vi "DalyLab_Oscilloscope_DAQ_v1.0.vi"() -> ()   [LabVIEW 2017]
uses:
  897ebd14-b167-4137-bf33-77dfcdb94355.vi
  <vilib>/Utility/file.llb/Write Delimited Spreadsheet (DBL).vi
  <instrlib>/Keysight InfiniiVision/Keysight InfiniiVision.lvlib
panel:
  in  "Tab Control":T1(tab)
  in  "Frequency Sweep":bool
  out "SWEEP IN PROGRESS":bool
  in  "Amplitude (Vpp)":dbl=5.0 format="%#_13g"
  in  "Initial Frequency (Hz)":dbl=20000.0 format="%#_13g"
  in  "Stop Frequency (Hz)":dbl=30000.0 format="%#_13g"
  in  "Freq. Increments (Hz)":dbl=1000.0 format="%#_13g"
  in  "Acq. per Freq.":i32=1
  out "Sine Freq (Hz)":dbl format="%#_13g"
  in  "Delay (ms)":dbl=1000.0 format="%#_13g"
  in  "Pulse Generation":bool
  out "PULSING IN PROGRESS":bool
  in  "Pulse Width (s)":dbl=1e-06 format="%#_13g"
  in  "Rate (pulse/second)":dbl=1.0 format="%#_13g"
  in  "Pulse Amplitude (V)":dbl=5.0 format="%#_13g"
  in  "Number of Pulses":i32=30
  in  "Acquisition":bool
  in  "Stop Acquisition":bool
  out "ACQUISITION IN PROGRESS":bool
  out "Channel 2":dbl[](graph)
  out "EVENT COUNTER":dbl
  out "Log":string caption="LOG"
  out "Channel 1":dbl[](graph)
  in  "Acq. Start Time (s)":dbl=-0.0008
  in  "Horizontal Scale (s/div)":dbl=0.0002
  in  "Channel 2 Atten.":dbl=1.0 format="%#_13g"
  in  "Channel 1 Atten.":dbl=1.0 format="%#_13g"
  in  "Channel 2 Offset (V)":dbl
  in  "Channel 2 Scale (V/div)":dbl=0.05
  in  "Channel 1 Offset (V)":dbl
  in  "Channel 1 Scale (V/div)":dbl=1.0
  in  "Trigger Edge Level (V)":dbl=0.05
  in  "Trigger Edge Source":u16(ring) items=["Channel1", "Channel2"]
  in  "Test Operator":string
  out "File Path":path
  in  "File Name":string
  in  "Save Directory":path
  in  "Oscilloscope VISA address":string="USB0::0x0957::0x1797::MY56271380::0::INSTR" caption="Oscilloscope VISA Address"
  in  "Waveform Size":i32=50000
  out "Test Type":i32
  # "OSCILLOSCOPE CONFIGURATION"
  # "TESTING"
  # "SETUP"
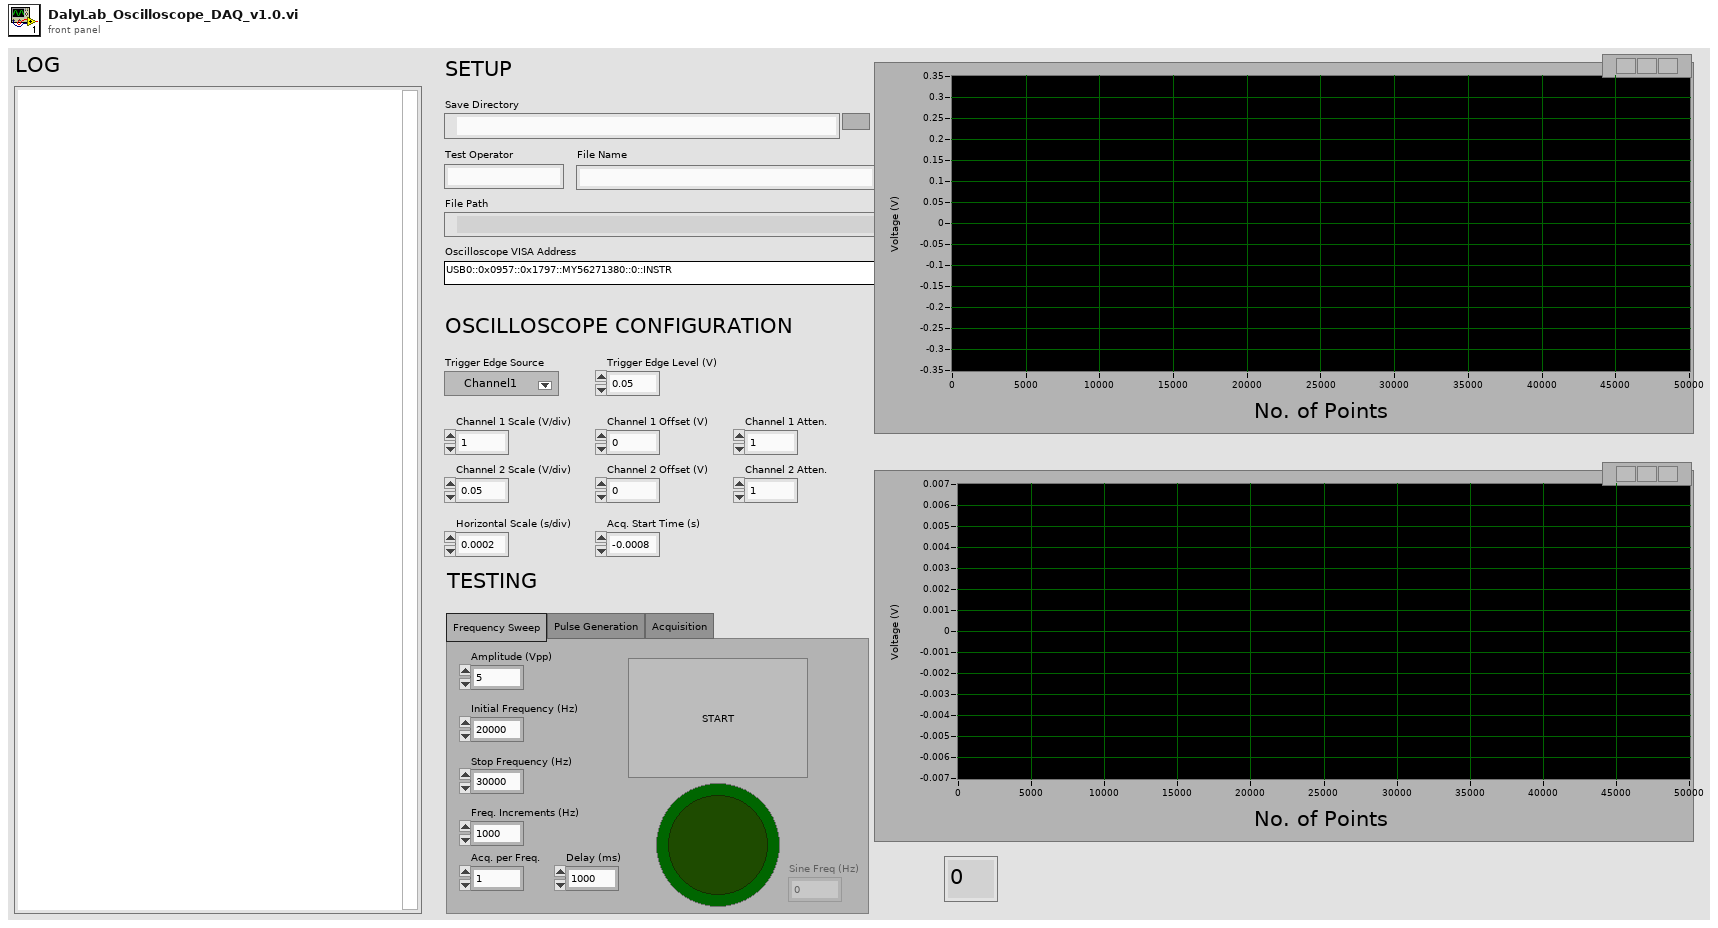
[diagram p1: front panel]
types:
  T1 = enum32{"Frequency Sweep", "Pulse Generation", "Acquisition"}
  T2 = enum16{"open", "replace", "create", "open or create", "replace or create", "replace or create with confirmation"}
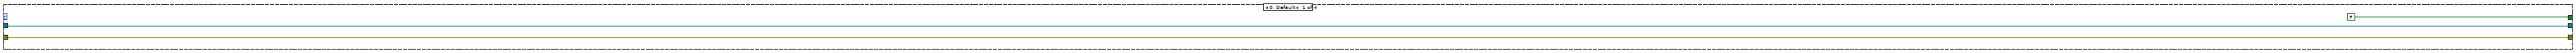
[diagram p5: hidden frame]
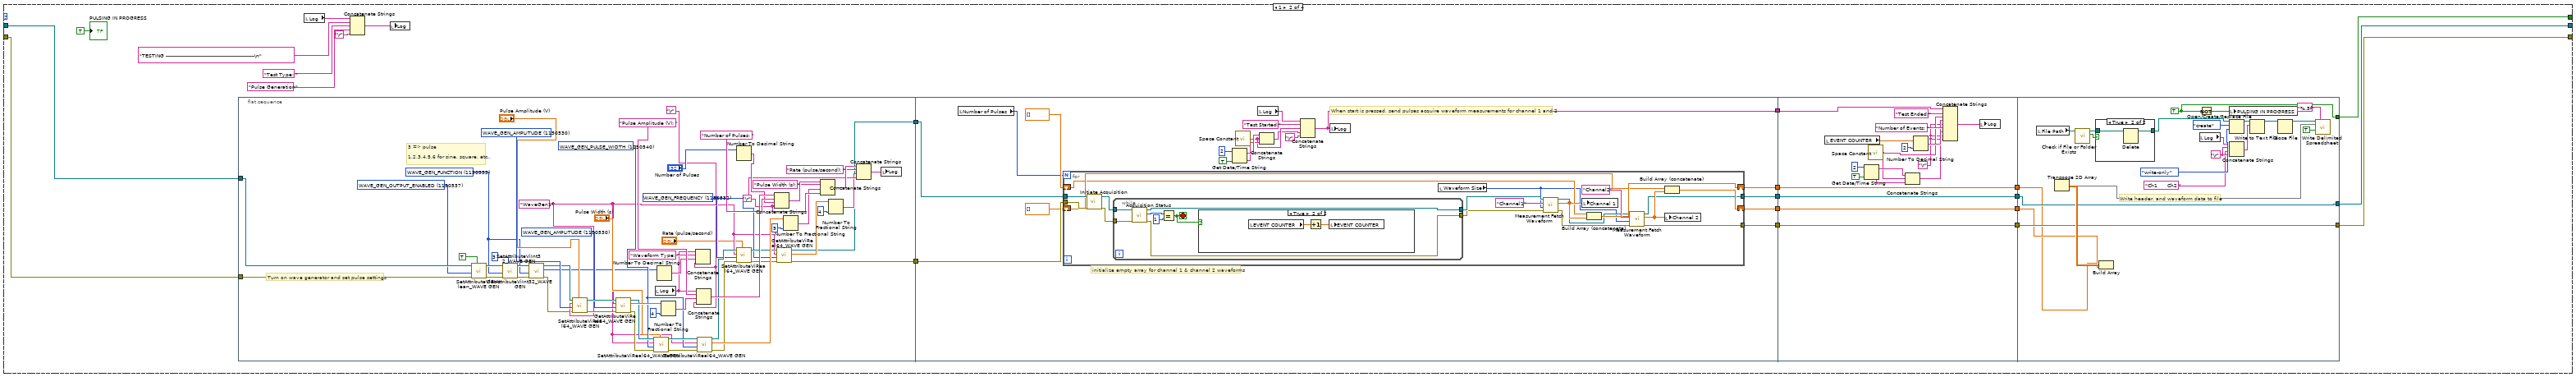
[diagram p6: hidden frame]
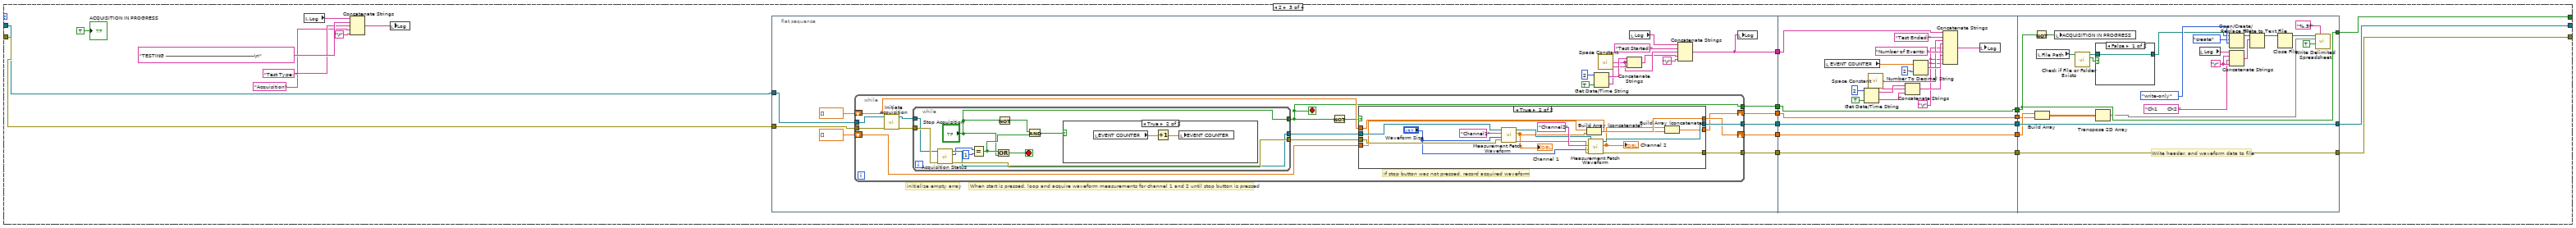
[diagram p9: hidden frame]
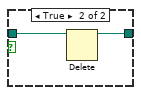
[diagram p12: hidden frame]
diagram:
  w2 = u32 1150537 items=["ARBITRARY_INTERPOLATION"=1150411, "MODULATION_ENABLED"=1150554, "TRACKING_AMPLITUDE"=1150527, "TRACKING_ENABLED"=1150526, "TRACKING_FREQUENCY"=1150528, "WAVE_GEN_ARBITRARY_INTERPOLATION"=1150543, "WAVE_GEN_OUTPUT_ENABLED"=1150537, "WAVE_GEN_OUTPUT_INVERTED"=1150545] ("AttributeID")
  w9 = "\r"
  w18 = "\r"
  w22 = "\r"
  w50 = u32 1250004 items=["ACQUISITION_START_TIME"=1250109, "CHANNEL_PROBE_SKEW"=1150030, "CHANNEL_SCALE"=1150032, "EXTERNAL_PROBE_ATTENUATION"=1150012, "EXTERNAL_RANGE"=1150015, "GLITCH_WIDTH"=1250401, "HORZ_TIME_PER_RECORD"=1250007, "INPUT_IMPEDANCE"=1250103, "INTEGRATE_INPUT_OFFSET"=1150360, "MAX_INPUT_FREQUENCY"=1250006, "MEAS_HIGH_REF"=1250607, "MEAS_LOW_REF"=1250608, "MEAS_MID_REF"=1250609, "PROBE_ATTENUATION"=1250004, "RUNT_HIGH_THRESHOLD"=1250301, "RUNT_LOW_THRESHOLD"=1250302, "TIMEBASE_HORIZONTAL_SCALE"=1150111, "TIMEBASE_WINDOW_HORIZONTAL_SCALE"=1150115, "TIMEBASE_WINDOW_POSITION"=1150113, "TIMEBASE_WINDOW_RANGE"=1150114, "TRIGGER_DELAY_TIME"=1150265, "TRIGGER_EDGE_BURST_IDLE_TIME"=1150248, "TRIGGER_GLITCH_LEVEL"=1150134, "TRIGGER_HOLDOFF"=1250016, "TRIGGER_LEVEL"=1250017, "TRIGGER_PATTERN_MAX_DURATION"=1150166, "TRIGGER_PATTERN_MIN_WIDTH"=1150158, "TRIGGER_RUNT_QUALIFIER_TIME"=1150191, "TRIGGER_SETUP_AND_HOLD_HOLD_TIME"=1150251, "TRIGGER_SETUP_AND_HOLD_SETUP_TIME"=1150252, "TRIGGER_TRANSITION_QUALIFIER_TIME"=1150257, "TRIGGER_TRANSITION_THRESHOLD_HIGH"=1150428, "TRIGGER_TRANSITION_THRESHOLD_LOW"=1150429, "TRIGGER_WIDTH_THRESHOLD_HIGH"=1150198, "TRIGGER_WIDTH_THRESHOLD_LOW"=1150199, "VERTICAL_OFFSET"=1250002, "VERTICAL_RANGE"=1250001, "WIDTH_HIGH_THRESHOLD"=1250502, "WIDTH_LOW_THRESHOLD"=1250501] ("AttributeID")
  w51 = "Channel2"
  w70 = "Channel1"
  w69 = u32 1250004 items=["ACQUISITION_START_TIME"=1250109, "CHANNEL_PROBE_SKEW"=1150030, "CHANNEL_SCALE"=1150032, "EXTERNAL_PROBE_ATTENUATION"=1150012, "EXTERNAL_RANGE"=1150015, "GLITCH_WIDTH"=1250401, "HORZ_TIME_PER_RECORD"=1250007, "INPUT_IMPEDANCE"=1250103, "INTEGRATE_INPUT_OFFSET"=1150360, "MAX_INPUT_FREQUENCY"=1250006, "MEAS_HIGH_REF"=1250607, "MEAS_LOW_REF"=1250608, "MEAS_MID_REF"=1250609, "PROBE_ATTENUATION"=1250004, "RUNT_HIGH_THRESHOLD"=1250301, "RUNT_LOW_THRESHOLD"=1250302, "TIMEBASE_HORIZONTAL_SCALE"=1150111, "TIMEBASE_WINDOW_HORIZONTAL_SCALE"=1150115, "TIMEBASE_WINDOW_POSITION"=1150113, "TIMEBASE_WINDOW_RANGE"=1150114, "TRIGGER_DELAY_TIME"=1150265, "TRIGGER_EDGE_BURST_IDLE_TIME"=1150248, "TRIGGER_GLITCH_LEVEL"=1150134, "TRIGGER_HOLDOFF"=1250016, "TRIGGER_LEVEL"=1250017, "TRIGGER_PATTERN_MAX_DURATION"=1150166, "TRIGGER_PATTERN_MIN_WIDTH"=1150158, "TRIGGER_RUNT_QUALIFIER_TIME"=1150191, "TRIGGER_SETUP_AND_HOLD_HOLD_TIME"=1150251, "TRIGGER_SETUP_AND_HOLD_SETUP_TIME"=1150252, "TRIGGER_TRANSITION_QUALIFIER_TIME"=1150257, "TRIGGER_TRANSITION_THRESHOLD_HIGH"=1150428, "TRIGGER_TRANSITION_THRESHOLD_LOW"=1150429, "TRIGGER_WIDTH_THRESHOLD_HIGH"=1150198, "TRIGGER_WIDTH_THRESHOLD_LOW"=1150199, "VERTICAL_OFFSET"=1250002, "VERTICAL_RANGE"=1250001, "WIDTH_HIGH_THRESHOLD"=1250502, "WIDTH_LOW_THRESHOLD"=1250501] ("AttributeID")
  w81 = "Channel2"
  w84 = u32 1250002 items=["ACQUISITION_START_TIME"=1250109, "CHANNEL_PROBE_SKEW"=1150030, "CHANNEL_SCALE"=1150032, "EXTERNAL_PROBE_ATTENUATION"=1150012, "EXTERNAL_RANGE"=1150015, "GLITCH_WIDTH"=1250401, "HORZ_TIME_PER_RECORD"=1250007, "INPUT_IMPEDANCE"=1250103, "INTEGRATE_INPUT_OFFSET"=1150360, "MAX_INPUT_FREQUENCY"=1250006, "MEAS_HIGH_REF"=1250607, "MEAS_LOW_REF"=1250608, "MEAS_MID_REF"=1250609, "PROBE_ATTENUATION"=1250004, "RUNT_HIGH_THRESHOLD"=1250301, "RUNT_LOW_THRESHOLD"=1250302, "TIMEBASE_HORIZONTAL_SCALE"=1150111, "TIMEBASE_WINDOW_HORIZONTAL_SCALE"=1150115, "TIMEBASE_WINDOW_POSITION"=1150113, "TIMEBASE_WINDOW_RANGE"=1150114, "TRIGGER_DELAY_TIME"=1150265, "TRIGGER_EDGE_BURST_IDLE_TIME"=1150248, "TRIGGER_GLITCH_LEVEL"=1150134, "TRIGGER_HOLDOFF"=1250016, "TRIGGER_LEVEL"=1250017, "TRIGGER_PATTERN_MAX_DURATION"=1150166, "TRIGGER_PATTERN_MIN_WIDTH"=1150158, "TRIGGER_RUNT_QUALIFIER_TIME"=1150191, "TRIGGER_SETUP_AND_HOLD_HOLD_TIME"=1150251, "TRIGGER_SETUP_AND_HOLD_SETUP_TIME"=1150252, "TRIGGER_TRANSITION_QUALIFIER_TIME"=1150257, "TRIGGER_TRANSITION_THRESHOLD_HIGH"=1150428, "TRIGGER_TRANSITION_THRESHOLD_LOW"=1150429, "TRIGGER_WIDTH_THRESHOLD_HIGH"=1150198, "TRIGGER_WIDTH_THRESHOLD_LOW"=1150199, "VERTICAL_OFFSET"=1250002, "VERTICAL_RANGE"=1250001, "WIDTH_HIGH_THRESHOLD"=1250502, "WIDTH_LOW_THRESHOLD"=1250501] ("AttributeID")
  w85 = u32 1250002 items=["ACQUISITION_START_TIME"=1250109, "CHANNEL_PROBE_SKEW"=1150030, "CHANNEL_SCALE"=1150032, "EXTERNAL_PROBE_ATTENUATION"=1150012, "EXTERNAL_RANGE"=1150015, "GLITCH_WIDTH"=1250401, "HORZ_TIME_PER_RECORD"=1250007, "INPUT_IMPEDANCE"=1250103, "INTEGRATE_INPUT_OFFSET"=1150360, "MAX_INPUT_FREQUENCY"=1250006, "MEAS_HIGH_REF"=1250607, "MEAS_LOW_REF"=1250608, "MEAS_MID_REF"=1250609, "PROBE_ATTENUATION"=1250004, "RUNT_HIGH_THRESHOLD"=1250301, "RUNT_LOW_THRESHOLD"=1250302, "TIMEBASE_HORIZONTAL_SCALE"=1150111, "TIMEBASE_WINDOW_HORIZONTAL_SCALE"=1150115, "TIMEBASE_WINDOW_POSITION"=1150113, "TIMEBASE_WINDOW_RANGE"=1150114, "TRIGGER_DELAY_TIME"=1150265, "TRIGGER_EDGE_BURST_IDLE_TIME"=1150248, "TRIGGER_GLITCH_LEVEL"=1150134, "TRIGGER_HOLDOFF"=1250016, "TRIGGER_LEVEL"=1250017, "TRIGGER_PATTERN_MAX_DURATION"=1150166, "TRIGGER_PATTERN_MIN_WIDTH"=1150158, "TRIGGER_RUNT_QUALIFIER_TIME"=1150191, "TRIGGER_SETUP_AND_HOLD_HOLD_TIME"=1150251, "TRIGGER_SETUP_AND_HOLD_SETUP_TIME"=1150252, "TRIGGER_TRANSITION_QUALIFIER_TIME"=1150257, "TRIGGER_TRANSITION_THRESHOLD_HIGH"=1150428, "TRIGGER_TRANSITION_THRESHOLD_LOW"=1150429, "TRIGGER_WIDTH_THRESHOLD_HIGH"=1150198, "TRIGGER_WIDTH_THRESHOLD_LOW"=1150199, "VERTICAL_OFFSET"=1250002, "VERTICAL_RANGE"=1250001, "WIDTH_HIGH_THRESHOLD"=1250502, "WIDTH_LOW_THRESHOLD"=1250501] ("AttributeID")
  w103 = u32 1150032 items=["ACQUISITION_SEGMENTEDMEMORY_TIME_TAG"=1150140, "ACQUISITION_START_TIME"=1250109, "CHANNEL_PROBE_SKEW"=1150030, "CHANNEL_SCALE"=1150032, "DVM_CURRENT"=1150440, "DVM_FREQUENCY"=1150442, "EXTERNAL_PROBE_ATTENUATION"=1150012, "EXTERNAL_PROBE_SENSE"=1150013, "EXTERNAL_RANGE"=1150015, "GLITCH_WIDTH"=1250401, "HORZ_SAMPLE_RATE"=1250010, "HORZ_TIME_PER_RECORD"=1250007, "INPUT_IMPEDANCE"=1250103, "INTEGRATE_INPUT_OFFSET"=1150360, "MAX_INPUT_FREQUENCY"=1250006, "MEAS_HIGH_REF"=1250607, "MEAS_LOW_REF"=1250608, "MEAS_MID_REF"=1250609, "PROBE_ATTENUATION"=1250004, "PROBE_SENSE_VALUE"=1250108, "RUNT_HIGH_THRESHOLD"=1250301, "RUNT_LOW_THRESHOLD"=1250302, "TIMEBASE_HORIZONTAL_SCALE"=1150111, "TIMEBASE_WINDOW_HORIZONTAL_SCALE"=1150115, "TIMEBASE_WINDOW_POSITION"=1150113, "TIMEBASE_WINDOW_RANGE"=1150114, "TRIGGER_DELAY_TIME"=1150265, "TRIGGER_EDGE_BURST_IDLE_TIME"=1150248, "TRIGGER_GLITCH_LEVEL"=1150134, "TRIGGER_HOLDOFF"=1250016, "TRIGGER_LEVEL"=1250017, "TRIGGER_PATTERN_MAX_DURATION"=1150166, "TRIGGER_PATTERN_MIN_WIDTH"=1150158, "TRIGGER_RUNT_QUALIFIER_TIME"=1150191, "TRIGGER_SETUP_AND_HOLD_HOLD_TIME"=1150251, "TRIGGER_SETUP_AND_HOLD_SETUP_TIME"=1150252, "TRIGGER_TRANSITION_QUALIFIER_TIME"=1150257, "TRIGGER_TRANSITION_THRESHOLD_HIGH"=1150428, "TRIGGER_TRANSITION_THRESHOLD_LOW"=1150429, "TRIGGER_WIDTH_THRESHOLD_HIGH"=1150198, "TRIGGER_WIDTH_THRESHOLD_LOW"=1150199, "VERTICAL_OFFSET"=1250002, "VERTICAL_RANGE"=1250001, "WAVEFORM_X_INCREMENT"=1150143, "WAVEFORM_X_ORIGIN"=1150147, "WAVEFORM_Y_INCREMENT"=1150144, "WAVEFORM_Y_ORIGIN"=1150148, "WIDTH_HIGH_THRESHOLD"=1250502, "WIDTH_LOW_THRESHOLD"=1250501] ("AttributeID")
  w104 = u32 1150032 items=["ACQUISITION_SEGMENTEDMEMORY_TIME_TAG"=1150140, "ACQUISITION_START_TIME"=1250109, "CHANNEL_PROBE_SKEW"=1150030, "CHANNEL_SCALE"=1150032, "DVM_CURRENT"=1150440, "DVM_FREQUENCY"=1150442, "EXTERNAL_PROBE_ATTENUATION"=1150012, "EXTERNAL_PROBE_SENSE"=1150013, "EXTERNAL_RANGE"=1150015, "GLITCH_WIDTH"=1250401, "HORZ_SAMPLE_RATE"=1250010, "HORZ_TIME_PER_RECORD"=1250007, "INPUT_IMPEDANCE"=1250103, "INTEGRATE_INPUT_OFFSET"=1150360, "MAX_INPUT_FREQUENCY"=1250006, "MEAS_HIGH_REF"=1250607, "MEAS_LOW_REF"=1250608, "MEAS_MID_REF"=1250609, "PROBE_ATTENUATION"=1250004, "PROBE_SENSE_VALUE"=1250108, "RUNT_HIGH_THRESHOLD"=1250301, "RUNT_LOW_THRESHOLD"=1250302, "TIMEBASE_HORIZONTAL_SCALE"=1150111, "TIMEBASE_WINDOW_HORIZONTAL_SCALE"=1150115, "TIMEBASE_WINDOW_POSITION"=1150113, "TIMEBASE_WINDOW_RANGE"=1150114, "TRIGGER_DELAY_TIME"=1150265, "TRIGGER_EDGE_BURST_IDLE_TIME"=1150248, "TRIGGER_GLITCH_LEVEL"=1150134, "TRIGGER_HOLDOFF"=1250016, "TRIGGER_LEVEL"=1250017, "TRIGGER_PATTERN_MAX_DURATION"=1150166, "TRIGGER_PATTERN_MIN_WIDTH"=1150158, "TRIGGER_RUNT_QUALIFIER_TIME"=1150191, "TRIGGER_SETUP_AND_HOLD_HOLD_TIME"=1150251, "TRIGGER_SETUP_AND_HOLD_SETUP_TIME"=1150252, "TRIGGER_TRANSITION_QUALIFIER_TIME"=1150257, "TRIGGER_TRANSITION_THRESHOLD_HIGH"=1150428, "TRIGGER_TRANSITION_THRESHOLD_LOW"=1150429, "TRIGGER_WIDTH_THRESHOLD_HIGH"=1150198, "TRIGGER_WIDTH_THRESHOLD_LOW"=1150199, "VERTICAL_OFFSET"=1250002, "VERTICAL_RANGE"=1250001, "WAVEFORM_X_INCREMENT"=1150143, "WAVEFORM_X_ORIGIN"=1150147, "WAVEFORM_Y_INCREMENT"=1150144, "WAVEFORM_Y_ORIGIN"=1150148, "WIDTH_HIGH_THRESHOLD"=1250502, "WIDTH_LOW_THRESHOLD"=1250501] ("AttributeID")
  w102 = "Channel2"
  w28 = FALSE
  w119 = u32 1250109 items=["ACQUISITION_START_TIME"=1250109, "CHANNEL_PROBE_SKEW"=1150030, "CHANNEL_SCALE"=1150032, "EXTERNAL_PROBE_ATTENUATION"=1150012, "EXTERNAL_RANGE"=1150015, "GLITCH_WIDTH"=1250401, "HORZ_TIME_PER_RECORD"=1250007, "INPUT_IMPEDANCE"=1250103, "INTEGRATE_INPUT_OFFSET"=1150360, "MAX_INPUT_FREQUENCY"=1250006, "MEAS_HIGH_REF"=1250607, "MEAS_LOW_REF"=1250608, "MEAS_MID_REF"=1250609, "PROBE_ATTENUATION"=1250004, "RUNT_HIGH_THRESHOLD"=1250301, "RUNT_LOW_THRESHOLD"=1250302, "TIMEBASE_HORIZONTAL_SCALE"=1150111, "TIMEBASE_WINDOW_HORIZONTAL_SCALE"=1150115, "TIMEBASE_WINDOW_POSITION"=1150113, "TIMEBASE_WINDOW_RANGE"=1150114, "TRIGGER_DELAY_TIME"=1150265, "TRIGGER_EDGE_BURST_IDLE_TIME"=1150248, "TRIGGER_GLITCH_LEVEL"=1150134, "TRIGGER_HOLDOFF"=1250016, "TRIGGER_LEVEL"=1250017, "TRIGGER_PATTERN_MAX_DURATION"=1150166, "TRIGGER_PATTERN_MIN_WIDTH"=1150158, "TRIGGER_RUNT_QUALIFIER_TIME"=1150191, "TRIGGER_SETUP_AND_HOLD_HOLD_TIME"=1150251, "TRIGGER_SETUP_AND_HOLD_SETUP_TIME"=1150252, "TRIGGER_TRANSITION_QUALIFIER_TIME"=1150257, "TRIGGER_TRANSITION_THRESHOLD_HIGH"=1150428, "TRIGGER_TRANSITION_THRESHOLD_LOW"=1150429, "TRIGGER_WIDTH_THRESHOLD_HIGH"=1150198, "TRIGGER_WIDTH_THRESHOLD_LOW"=1150199, "VERTICAL_OFFSET"=1250002, "VERTICAL_RANGE"=1250001, "WIDTH_HIGH_THRESHOLD"=1250502, "WIDTH_LOW_THRESHOLD"=1250501] ("AttributeID")
  w121 = u32 1250109 items=["ACQUISITION_START_TIME"=1250109, "CHANNEL_PROBE_SKEW"=1150030, "CHANNEL_SCALE"=1150032, "EXTERNAL_PROBE_ATTENUATION"=1150012, "EXTERNAL_RANGE"=1150015, "GLITCH_WIDTH"=1250401, "HORZ_TIME_PER_RECORD"=1250007, "INPUT_IMPEDANCE"=1250103, "INTEGRATE_INPUT_OFFSET"=1150360, "MAX_INPUT_FREQUENCY"=1250006, "MEAS_HIGH_REF"=1250607, "MEAS_LOW_REF"=1250608, "MEAS_MID_REF"=1250609, "PROBE_ATTENUATION"=1250004, "RUNT_HIGH_THRESHOLD"=1250301, "RUNT_LOW_THRESHOLD"=1250302, "TIMEBASE_HORIZONTAL_SCALE"=1150111, "TIMEBASE_WINDOW_HORIZONTAL_SCALE"=1150115, "TIMEBASE_WINDOW_POSITION"=1150113, "TIMEBASE_WINDOW_RANGE"=1150114, "TRIGGER_DELAY_TIME"=1150265, "TRIGGER_EDGE_BURST_IDLE_TIME"=1150248, "TRIGGER_GLITCH_LEVEL"=1150134, "TRIGGER_HOLDOFF"=1250016, "TRIGGER_LEVEL"=1250017, "TRIGGER_PATTERN_MAX_DURATION"=1150166, "TRIGGER_PATTERN_MIN_WIDTH"=1150158, "TRIGGER_RUNT_QUALIFIER_TIME"=1150191, "TRIGGER_SETUP_AND_HOLD_HOLD_TIME"=1150251, "TRIGGER_SETUP_AND_HOLD_SETUP_TIME"=1150252, "TRIGGER_TRANSITION_QUALIFIER_TIME"=1150257, "TRIGGER_TRANSITION_THRESHOLD_HIGH"=1150428, "TRIGGER_TRANSITION_THRESHOLD_LOW"=1150429, "TRIGGER_WIDTH_THRESHOLD_HIGH"=1150198, "TRIGGER_WIDTH_THRESHOLD_LOW"=1150199, "VERTICAL_OFFSET"=1250002, "VERTICAL_RANGE"=1250001, "WIDTH_HIGH_THRESHOLD"=1250502, "WIDTH_LOW_THRESHOLD"=1250501] ("AttributeID")
  w122 = u32 1150111 items=["ACQUISITION_SEGMENTEDMEMORY_TIME_TAG"=1150140, "ACQUISITION_START_TIME"=1250109, "CHANNEL_PROBE_SKEW"=1150030, "CHANNEL_SCALE"=1150032, "DVM_CURRENT"=1150440, "DVM_FREQUENCY"=1150442, "EXTERNAL_PROBE_ATTENUATION"=1150012, "EXTERNAL_PROBE_SENSE"=1150013, "EXTERNAL_RANGE"=1150015, "GLITCH_WIDTH"=1250401, "HORZ_SAMPLE_RATE"=1250010, "HORZ_TIME_PER_RECORD"=1250007, "INPUT_IMPEDANCE"=1250103, "INTEGRATE_INPUT_OFFSET"=1150360, "MAX_INPUT_FREQUENCY"=1250006, "MEAS_HIGH_REF"=1250607, "MEAS_LOW_REF"=1250608, "MEAS_MID_REF"=1250609, "PROBE_ATTENUATION"=1250004, "PROBE_SENSE_VALUE"=1250108, "RUNT_HIGH_THRESHOLD"=1250301, "RUNT_LOW_THRESHOLD"=1250302, "TIMEBASE_HORIZONTAL_SCALE"=1150111, "TIMEBASE_WINDOW_HORIZONTAL_SCALE"=1150115, "TIMEBASE_WINDOW_POSITION"=1150113, "TIMEBASE_WINDOW_RANGE"=1150114, "TRIGGER_DELAY_TIME"=1150265, "TRIGGER_EDGE_BURST_IDLE_TIME"=1150248, "TRIGGER_GLITCH_LEVEL"=1150134, "TRIGGER_HOLDOFF"=1250016, "TRIGGER_LEVEL"=1250017, "TRIGGER_PATTERN_MAX_DURATION"=1150166, "TRIGGER_PATTERN_MIN_WIDTH"=1150158, "TRIGGER_RUNT_QUALIFIER_TIME"=1150191, "TRIGGER_SETUP_AND_HOLD_HOLD_TIME"=1150251, "TRIGGER_SETUP_AND_HOLD_SETUP_TIME"=1150252, "TRIGGER_TRANSITION_QUALIFIER_TIME"=1150257, "TRIGGER_TRANSITION_THRESHOLD_HIGH"=1150428, "TRIGGER_TRANSITION_THRESHOLD_LOW"=1150429, "TRIGGER_WIDTH_THRESHOLD_HIGH"=1150198, "TRIGGER_WIDTH_THRESHOLD_LOW"=1150199, "VERTICAL_OFFSET"=1250002, "VERTICAL_RANGE"=1250001, "WAVEFORM_X_INCREMENT"=1150143, "WAVEFORM_X_ORIGIN"=1150147, "WAVEFORM_Y_INCREMENT"=1150144, "WAVEFORM_Y_ORIGIN"=1150148, "WIDTH_HIGH_THRESHOLD"=1250502, "WIDTH_LOW_THRESHOLD"=1250501] ("AttributeID")
  w125 = u32 1150111 items=["ACQUISITION_SEGMENTEDMEMORY_TIME_TAG"=1150140, "ACQUISITION_START_TIME"=1250109, "CHANNEL_PROBE_SKEW"=1150030, "CHANNEL_SCALE"=1150032, "DVM_CURRENT"=1150440, "DVM_FREQUENCY"=1150442, "EXTERNAL_PROBE_ATTENUATION"=1150012, "EXTERNAL_PROBE_SENSE"=1150013, "EXTERNAL_RANGE"=1150015, "GLITCH_WIDTH"=1250401, "HORZ_SAMPLE_RATE"=1250010, "HORZ_TIME_PER_RECORD"=1250007, "INPUT_IMPEDANCE"=1250103, "INTEGRATE_INPUT_OFFSET"=1150360, "MAX_INPUT_FREQUENCY"=1250006, "MEAS_HIGH_REF"=1250607, "MEAS_LOW_REF"=1250608, "MEAS_MID_REF"=1250609, "PROBE_ATTENUATION"=1250004, "PROBE_SENSE_VALUE"=1250108, "RUNT_HIGH_THRESHOLD"=1250301, "RUNT_LOW_THRESHOLD"=1250302, "TIMEBASE_HORIZONTAL_SCALE"=1150111, "TIMEBASE_WINDOW_HORIZONTAL_SCALE"=1150115, "TIMEBASE_WINDOW_POSITION"=1150113, "TIMEBASE_WINDOW_RANGE"=1150114, "TRIGGER_DELAY_TIME"=1150265, "TRIGGER_EDGE_BURST_IDLE_TIME"=1150248, "TRIGGER_GLITCH_LEVEL"=1150134, "TRIGGER_HOLDOFF"=1250016, "TRIGGER_LEVEL"=1250017, "TRIGGER_PATTERN_MAX_DURATION"=1150166, "TRIGGER_PATTERN_MIN_WIDTH"=1150158, "TRIGGER_RUNT_QUALIFIER_TIME"=1150191, "TRIGGER_SETUP_AND_HOLD_HOLD_TIME"=1150251, "TRIGGER_SETUP_AND_HOLD_SETUP_TIME"=1150252, "TRIGGER_TRANSITION_QUALIFIER_TIME"=1150257, "TRIGGER_TRANSITION_THRESHOLD_HIGH"=1150428, "TRIGGER_TRANSITION_THRESHOLD_LOW"=1150429, "TRIGGER_WIDTH_THRESHOLD_HIGH"=1150198, "TRIGGER_WIDTH_THRESHOLD_LOW"=1150199, "VERTICAL_OFFSET"=1250002, "VERTICAL_RANGE"=1250001, "WAVEFORM_X_INCREMENT"=1150143, "WAVEFORM_X_ORIGIN"=1150147, "WAVEFORM_Y_INCREMENT"=1150144, "WAVEFORM_Y_ORIGIN"=1150148, "WIDTH_HIGH_THRESHOLD"=1250502, "WIDTH_LOW_THRESHOLD"=1250501] ("AttributeID")
  w126 = "Channel1"
  w131 = u32 1250002 items=["ACQUISITION_START_TIME"=1250109, "CHANNEL_PROBE_SKEW"=1150030, "CHANNEL_SCALE"=1150032, "EXTERNAL_PROBE_ATTENUATION"=1150012, "EXTERNAL_RANGE"=1150015, "GLITCH_WIDTH"=1250401, "HORZ_TIME_PER_RECORD"=1250007, "INPUT_IMPEDANCE"=1250103, "INTEGRATE_INPUT_OFFSET"=1150360, "MAX_INPUT_FREQUENCY"=1250006, "MEAS_HIGH_REF"=1250607, "MEAS_LOW_REF"=1250608, "MEAS_MID_REF"=1250609, "PROBE_ATTENUATION"=1250004, "RUNT_HIGH_THRESHOLD"=1250301, "RUNT_LOW_THRESHOLD"=1250302, "TIMEBASE_HORIZONTAL_SCALE"=1150111, "TIMEBASE_WINDOW_HORIZONTAL_SCALE"=1150115, "TIMEBASE_WINDOW_POSITION"=1150113, "TIMEBASE_WINDOW_RANGE"=1150114, "TRIGGER_DELAY_TIME"=1150265, "TRIGGER_EDGE_BURST_IDLE_TIME"=1150248, "TRIGGER_GLITCH_LEVEL"=1150134, "TRIGGER_HOLDOFF"=1250016, "TRIGGER_LEVEL"=1250017, "TRIGGER_PATTERN_MAX_DURATION"=1150166, "TRIGGER_PATTERN_MIN_WIDTH"=1150158, "TRIGGER_RUNT_QUALIFIER_TIME"=1150191, "TRIGGER_SETUP_AND_HOLD_HOLD_TIME"=1150251, "TRIGGER_SETUP_AND_HOLD_SETUP_TIME"=1150252, "TRIGGER_TRANSITION_QUALIFIER_TIME"=1150257, "TRIGGER_TRANSITION_THRESHOLD_HIGH"=1150428, "TRIGGER_TRANSITION_THRESHOLD_LOW"=1150429, "TRIGGER_WIDTH_THRESHOLD_HIGH"=1150198, "TRIGGER_WIDTH_THRESHOLD_LOW"=1150199, "VERTICAL_OFFSET"=1250002, "VERTICAL_RANGE"=1250001, "WIDTH_HIGH_THRESHOLD"=1250502, "WIDTH_LOW_THRESHOLD"=1250501] ("AttributeID")
  w132 = u32 1250002 items=["ACQUISITION_START_TIME"=1250109, "CHANNEL_PROBE_SKEW"=1150030, "CHANNEL_SCALE"=1150032, "EXTERNAL_PROBE_ATTENUATION"=1150012, "EXTERNAL_RANGE"=1150015, "GLITCH_WIDTH"=1250401, "HORZ_TIME_PER_RECORD"=1250007, "INPUT_IMPEDANCE"=1250103, "INTEGRATE_INPUT_OFFSET"=1150360, "MAX_INPUT_FREQUENCY"=1250006, "MEAS_HIGH_REF"=1250607, "MEAS_LOW_REF"=1250608, "MEAS_MID_REF"=1250609, "PROBE_ATTENUATION"=1250004, "RUNT_HIGH_THRESHOLD"=1250301, "RUNT_LOW_THRESHOLD"=1250302, "TIMEBASE_HORIZONTAL_SCALE"=1150111, "TIMEBASE_WINDOW_HORIZONTAL_SCALE"=1150115, "TIMEBASE_WINDOW_POSITION"=1150113, "TIMEBASE_WINDOW_RANGE"=1150114, "TRIGGER_DELAY_TIME"=1150265, "TRIGGER_EDGE_BURST_IDLE_TIME"=1150248, "TRIGGER_GLITCH_LEVEL"=1150134, "TRIGGER_HOLDOFF"=1250016, "TRIGGER_LEVEL"=1250017, "TRIGGER_PATTERN_MAX_DURATION"=1150166, "TRIGGER_PATTERN_MIN_WIDTH"=1150158, "TRIGGER_RUNT_QUALIFIER_TIME"=1150191, "TRIGGER_SETUP_AND_HOLD_HOLD_TIME"=1150251, "TRIGGER_SETUP_AND_HOLD_SETUP_TIME"=1150252, "TRIGGER_TRANSITION_QUALIFIER_TIME"=1150257, "TRIGGER_TRANSITION_THRESHOLD_HIGH"=1150428, "TRIGGER_TRANSITION_THRESHOLD_LOW"=1150429, "TRIGGER_WIDTH_THRESHOLD_HIGH"=1150198, "TRIGGER_WIDTH_THRESHOLD_LOW"=1150199, "VERTICAL_OFFSET"=1250002, "VERTICAL_RANGE"=1250001, "WIDTH_HIGH_THRESHOLD"=1250502, "WIDTH_LOW_THRESHOLD"=1250501] ("AttributeID")
  w136 = u32 1150032 items=["ACQUISITION_SEGMENTEDMEMORY_TIME_TAG"=1150140, "ACQUISITION_START_TIME"=1250109, "CHANNEL_PROBE_SKEW"=1150030, "CHANNEL_SCALE"=1150032, "DVM_CURRENT"=1150440, "DVM_FREQUENCY"=1150442, "EXTERNAL_PROBE_ATTENUATION"=1150012, "EXTERNAL_PROBE_SENSE"=1150013, "EXTERNAL_RANGE"=1150015, "GLITCH_WIDTH"=1250401, "HORZ_SAMPLE_RATE"=1250010, "HORZ_TIME_PER_RECORD"=1250007, "INPUT_IMPEDANCE"=1250103, "INTEGRATE_INPUT_OFFSET"=1150360, "MAX_INPUT_FREQUENCY"=1250006, "MEAS_HIGH_REF"=1250607, "MEAS_LOW_REF"=1250608, "MEAS_MID_REF"=1250609, "PROBE_ATTENUATION"=1250004, "PROBE_SENSE_VALUE"=1250108, "RUNT_HIGH_THRESHOLD"=1250301, "RUNT_LOW_THRESHOLD"=1250302, "TIMEBASE_HORIZONTAL_SCALE"=1150111, "TIMEBASE_WINDOW_HORIZONTAL_SCALE"=1150115, "TIMEBASE_WINDOW_POSITION"=1150113, "TIMEBASE_WINDOW_RANGE"=1150114, "TRIGGER_DELAY_TIME"=1150265, "TRIGGER_EDGE_BURST_IDLE_TIME"=1150248, "TRIGGER_GLITCH_LEVEL"=1150134, "TRIGGER_HOLDOFF"=1250016, "TRIGGER_LEVEL"=1250017, "TRIGGER_PATTERN_MAX_DURATION"=1150166, "TRIGGER_PATTERN_MIN_WIDTH"=1150158, "TRIGGER_RUNT_QUALIFIER_TIME"=1150191, "TRIGGER_SETUP_AND_HOLD_HOLD_TIME"=1150251, "TRIGGER_SETUP_AND_HOLD_SETUP_TIME"=1150252, "TRIGGER_TRANSITION_QUALIFIER_TIME"=1150257, "TRIGGER_TRANSITION_THRESHOLD_HIGH"=1150428, "TRIGGER_TRANSITION_THRESHOLD_LOW"=1150429, "TRIGGER_WIDTH_THRESHOLD_HIGH"=1150198, "TRIGGER_WIDTH_THRESHOLD_LOW"=1150199, "VERTICAL_OFFSET"=1250002, "VERTICAL_RANGE"=1250001, "WAVEFORM_X_INCREMENT"=1150143, "WAVEFORM_X_ORIGIN"=1150147, "WAVEFORM_Y_INCREMENT"=1150144, "WAVEFORM_Y_ORIGIN"=1150148, "WIDTH_HIGH_THRESHOLD"=1250502, "WIDTH_LOW_THRESHOLD"=1250501] ("AttributeID")
  w137 = u32 1150032 items=["ACQUISITION_SEGMENTEDMEMORY_TIME_TAG"=1150140, "ACQUISITION_START_TIME"=1250109, "CHANNEL_PROBE_SKEW"=1150030, "CHANNEL_SCALE"=1150032, "DVM_CURRENT"=1150440, "DVM_FREQUENCY"=1150442, "EXTERNAL_PROBE_ATTENUATION"=1150012, "EXTERNAL_PROBE_SENSE"=1150013, "EXTERNAL_RANGE"=1150015, "GLITCH_WIDTH"=1250401, "HORZ_SAMPLE_RATE"=1250010, "HORZ_TIME_PER_RECORD"=1250007, "INPUT_IMPEDANCE"=1250103, "INTEGRATE_INPUT_OFFSET"=1150360, "MAX_INPUT_FREQUENCY"=1250006, "MEAS_HIGH_REF"=1250607, "MEAS_LOW_REF"=1250608, "MEAS_MID_REF"=1250609, "PROBE_ATTENUATION"=1250004, "PROBE_SENSE_VALUE"=1250108, "RUNT_HIGH_THRESHOLD"=1250301, "RUNT_LOW_THRESHOLD"=1250302, "TIMEBASE_HORIZONTAL_SCALE"=1150111, "TIMEBASE_WINDOW_HORIZONTAL_SCALE"=1150115, "TIMEBASE_WINDOW_POSITION"=1150113, "TIMEBASE_WINDOW_RANGE"=1150114, "TRIGGER_DELAY_TIME"=1150265, "TRIGGER_EDGE_BURST_IDLE_TIME"=1150248, "TRIGGER_GLITCH_LEVEL"=1150134, "TRIGGER_HOLDOFF"=1250016, "TRIGGER_LEVEL"=1250017, "TRIGGER_PATTERN_MAX_DURATION"=1150166, "TRIGGER_PATTERN_MIN_WIDTH"=1150158, "TRIGGER_RUNT_QUALIFIER_TIME"=1150191, "TRIGGER_SETUP_AND_HOLD_HOLD_TIME"=1150251, "TRIGGER_SETUP_AND_HOLD_SETUP_TIME"=1150252, "TRIGGER_TRANSITION_QUALIFIER_TIME"=1150257, "TRIGGER_TRANSITION_THRESHOLD_HIGH"=1150428, "TRIGGER_TRANSITION_THRESHOLD_LOW"=1150429, "TRIGGER_WIDTH_THRESHOLD_HIGH"=1150198, "TRIGGER_WIDTH_THRESHOLD_LOW"=1150199, "VERTICAL_OFFSET"=1250002, "VERTICAL_RANGE"=1250001, "WAVEFORM_X_INCREMENT"=1150143, "WAVEFORM_X_ORIGIN"=1150147, "WAVEFORM_Y_INCREMENT"=1150144, "WAVEFORM_Y_ORIGIN"=1150148, "WIDTH_HIGH_THRESHOLD"=1250502, "WIDTH_LOW_THRESHOLD"=1250501] ("AttributeID")
  w135 = "Channel1"
  w171 = u32 1250017 items=["ACQUISITION_START_TIME"=1250109, "CHANNEL_PROBE_SKEW"=1150030, "CHANNEL_SCALE"=1150032, "EXTERNAL_PROBE_ATTENUATION"=1150012, "EXTERNAL_RANGE"=1150015, "GLITCH_WIDTH"=1250401, "HORZ_TIME_PER_RECORD"=1250007, "INPUT_IMPEDANCE"=1250103, "INTEGRATE_INPUT_OFFSET"=1150360, "MAX_INPUT_FREQUENCY"=1250006, "MEAS_HIGH_REF"=1250607, "MEAS_LOW_REF"=1250608, "MEAS_MID_REF"=1250609, "PROBE_ATTENUATION"=1250004, "RUNT_HIGH_THRESHOLD"=1250301, "RUNT_LOW_THRESHOLD"=1250302, "TIMEBASE_HORIZONTAL_SCALE"=1150111, "TIMEBASE_WINDOW_HORIZONTAL_SCALE"=1150115, "TIMEBASE_WINDOW_POSITION"=1150113, "TIMEBASE_WINDOW_RANGE"=1150114, "TRIGGER_DELAY_TIME"=1150265, "TRIGGER_EDGE_BURST_IDLE_TIME"=1150248, "TRIGGER_GLITCH_LEVEL"=1150134, "TRIGGER_HOLDOFF"=1250016, "TRIGGER_LEVEL"=1250017, "TRIGGER_PATTERN_MAX_DURATION"=1150166, "TRIGGER_PATTERN_MIN_WIDTH"=1150158, "TRIGGER_RUNT_QUALIFIER_TIME"=1150191, "TRIGGER_SETUP_AND_HOLD_HOLD_TIME"=1150251, "TRIGGER_SETUP_AND_HOLD_SETUP_TIME"=1150252, "TRIGGER_TRANSITION_QUALIFIER_TIME"=1150257, "TRIGGER_TRANSITION_THRESHOLD_HIGH"=1150428, "TRIGGER_TRANSITION_THRESHOLD_LOW"=1150429, "TRIGGER_WIDTH_THRESHOLD_HIGH"=1150198, "TRIGGER_WIDTH_THRESHOLD_LOW"=1150199, "VERTICAL_OFFSET"=1250002, "VERTICAL_RANGE"=1250001, "WIDTH_HIGH_THRESHOLD"=1250502, "WIDTH_LOW_THRESHOLD"=1250501] ("AttributeID")
  w176 = u32 1250017 items=["ACQUISITION_START_TIME"=1250109, "CHANNEL_PROBE_SKEW"=1150030, "CHANNEL_SCALE"=1150032, "EXTERNAL_PROBE_ATTENUATION"=1150012, "EXTERNAL_RANGE"=1150015, "GLITCH_WIDTH"=1250401, "HORZ_TIME_PER_RECORD"=1250007, "INPUT_IMPEDANCE"=1250103, "INTEGRATE_INPUT_OFFSET"=1150360, "MAX_INPUT_FREQUENCY"=1250006, "MEAS_HIGH_REF"=1250607, "MEAS_LOW_REF"=1250608, "MEAS_MID_REF"=1250609, "PROBE_ATTENUATION"=1250004, "RUNT_HIGH_THRESHOLD"=1250301, "RUNT_LOW_THRESHOLD"=1250302, "TIMEBASE_HORIZONTAL_SCALE"=1150111, "TIMEBASE_WINDOW_HORIZONTAL_SCALE"=1150115, "TIMEBASE_WINDOW_POSITION"=1150113, "TIMEBASE_WINDOW_RANGE"=1150114, "TRIGGER_DELAY_TIME"=1150265, "TRIGGER_EDGE_BURST_IDLE_TIME"=1150248, "TRIGGER_GLITCH_LEVEL"=1150134, "TRIGGER_HOLDOFF"=1250016, "TRIGGER_LEVEL"=1250017, "TRIGGER_PATTERN_MAX_DURATION"=1150166, "TRIGGER_PATTERN_MIN_WIDTH"=1150158, "TRIGGER_RUNT_QUALIFIER_TIME"=1150191, "TRIGGER_SETUP_AND_HOLD_HOLD_TIME"=1150251, "TRIGGER_SETUP_AND_HOLD_SETUP_TIME"=1150252, "TRIGGER_TRANSITION_QUALIFIER_TIME"=1150257, "TRIGGER_TRANSITION_THRESHOLD_HIGH"=1150428, "TRIGGER_TRANSITION_THRESHOLD_LOW"=1150429, "TRIGGER_WIDTH_THRESHOLD_HIGH"=1150198, "TRIGGER_WIDTH_THRESHOLD_LOW"=1150199, "VERTICAL_OFFSET"=1250002, "VERTICAL_RANGE"=1250001, "WIDTH_HIGH_THRESHOLD"=1250502, "WIDTH_LOW_THRESHOLD"=1250501] ("AttributeID")
  w182 = u32 1250013 items=["CHANNEL_LABEL"=1150027, "CHANNEL_PROBEID"=1150029, "DIGITALCHANNEL_LABEL"=1150040, "DIGITALCHANNEL_THRESHOLD"=1150043, "DRIVER_SETUP"=1050007, "DVM_SOURCE"=1150444, "INSTRUMENT_FIRMWARE_REVISION"=1050510, "INSTRUMENT_MANUFACTURER"=1050511, "INSTRUMENT_MODEL"=1050512, "IO_RESOURCE_DESCRIPTOR"=1050304, "LOGICAL_NAME"=1050305, "SPECIFIC_DRIVER_DESCRIPTION"=1050514, "SPECIFIC_DRIVER_REVISION"=1050551, "SPECIFIC_DRIVER_VENDOR"=1050513, "STATISTICS_COUNT"=1150356, "SUPPORTED_INSTRUMENT_MODELS"=1050327, "SYSTEM_SERIAL_NUMBER"=1150021, "SYSTEM_SYSTEM_DATE"=1150020, "SYSTEM_TIME"=1150022, "TRIGGER_DELAY_ARMING_SOURCE"=1150264, "TRIGGER_OR_EDGE_PATTERN"=1150262, "TRIGGER_PATTERN_ANALOG_PATTERN"=1150193, "TRIGGER_PATTERN_DIGITAL_PATTERN"=1150194, "TRIGGER_SETUP_AND_HOLD_CLOCK_SOURCE"=1150253, "TRIGGER_SETUP_AND_HOLD_DATA_SOURCE"=1150254, "TRIGGER_SOURCE"=1250013, "TRIGGER_ZONE_SOURCE"=1150468, "VIEW"=1150142, "WAVEFORM_SOURCE"=1150091] ("AttributeID")
  w183 = u32 1250013 items=["CHANNEL_LABEL"=1150027, "CHANNEL_PROBEID"=1150029, "DIGITALCHANNEL_LABEL"=1150040, "DIGITALCHANNEL_THRESHOLD"=1150043, "DRIVER_SETUP"=1050007, "DVM_SOURCE"=1150444, "INSTRUMENT_FIRMWARE_REVISION"=1050510, "INSTRUMENT_MANUFACTURER"=1050511, "INSTRUMENT_MODEL"=1050512, "IO_RESOURCE_DESCRIPTOR"=1050304, "LOGICAL_NAME"=1050305, "SPECIFIC_DRIVER_DESCRIPTION"=1050514, "SPECIFIC_DRIVER_REVISION"=1050551, "SPECIFIC_DRIVER_VENDOR"=1050513, "STATISTICS_COUNT"=1150356, "SUPPORTED_INSTRUMENT_MODELS"=1050327, "SYSTEM_SERIAL_NUMBER"=1150021, "SYSTEM_SYSTEM_DATE"=1150020, "SYSTEM_TIME"=1150022, "TRIGGER_DELAY_ARMING_SOURCE"=1150264, "TRIGGER_OR_EDGE_PATTERN"=1150262, "TRIGGER_PATTERN_ANALOG_PATTERN"=1150193, "TRIGGER_PATTERN_DIGITAL_PATTERN"=1150194, "TRIGGER_SETUP_AND_HOLD_CLOCK_SOURCE"=1150253, "TRIGGER_SETUP_AND_HOLD_DATA_SOURCE"=1150254, "TRIGGER_SOURCE"=1250013, "TRIGGER_ZONE_SOURCE"=1150468, "VIEW"=1150142, "WAVEFORM_SOURCE"=1150091] ("AttributeID")
  w184 = u32 1250012 items=["AC_LINE_TRIGGER_SLOPE"=1250701, "ACQUISITION_SEGMENTEDMEMORY_INDEX"=1150139, "ACQUISITION_SEGMENTEDMEMORY_SEGMENT_COUNT"=1150138, "ACQUISITION_TYPE"=1250101, "CHANNEL_COUNT"=1050203, "CHANNEL_PROTECTION"=1150202, "CHANNEL_UNITS"=1150033, "DIGITALCHANNEL_COUNT"=1150038, "DIGITALCHANNEL_POSITION"=1150041, "DIGITALCHANNEL_SIZE"=1150042, "DVM_MODE"=1150443, "EXTERNAL_UNITS"=1150014, "GLITCH_CONDITION"=1250403, "GLITCH_POLARITY"=1250402, "HORZ_MIN_NUM_PTS"=1250009, "HORZ_RECORD_LENGTH"=1250008, "INTERPOLATION"=1250019, "NUM_AVERAGES"=1250104, "NUM_ENVELOPES"=1250105, "REFERENCE_SIGNAL"=1150433, "RUNT_POLARITY"=1250303, "SAMPLE_MODE"=1250106, "STATISTICS_FORMAT"=1150355, "STATUS_SERIAL_POLL"=1150019, "SYSTEM_IO_TIMEOUT"=1150607, "SYSTEM_PRECISION_RECORD_LENGTH"=1150589, "SYSTEM_TIMEOUT_MILLISECONDS"=1150023, "TIMEBASE_MODE"=1150107, "TIMEBASE_TIME_REFERENCE"=1150110, "TRIGGER_ACLINE_SLOPE"=1150556, "TRIGGER_COUPLING"=1250014, "TRIGGER_DELAY_ARMING_SLOPE"=1150263, "TRIGGER_DELAY_EDGE_COUNT"=1150267, "TRIGGER_DELAY_SLOPE"=1150266, "TRIGGER_EDGE_BURST_NTH_EDGE"=1150247, "TRIGGER_EDGE_BURST_SLOPE"=1150249, "TRIGGER_EDGE_REJECT_FILTER_TYPE"=1150135, "TRIGGER_MODIFIER"=1250102, "TRIGGER_PATTERN_CONDITION"=1150195, "TRIGGER_RUNT_CONDITION"=1150189, "TRIGGER_SETUP_AND_HOLD_SLOPE"=1150250, "TRIGGER_SLOPE"=1250018, "TRIGGER_TRANSITION_CONDITION"=1150255, "TRIGGER_TRANSITION_SLOPE"=1150256, "TRIGGER_TYPE"=1250012, "TRIGGER_TYPE_AG"=1150557, "TRIGGER_WIDTH_CONDITION"=1150197, "TRIGGER_WIDTH_POLARITY"=1150200, "VERTICAL_COUPLING"=1250003, "WAVEFORM_BYTE_ORDER"=1150085, "WAVEFORM_DATA_FORMAT"=1150086, "WAVEFORM_POINT_COUNT"=1150141, "WAVEFORM_POINT_MODE"=1150087, "WAVEFORM_SUB_SOOURCE"=1150609, "WAVEFORM_X_REFERENCE"=1150145, "WAVEFORM_Y_REFERENCE"=1150146, "WIDTH_CONDITION"=1250504, "WIDTH_POLARITY"=1250503] ("AttributeID")
  w188 = u32 1250012 items=["AC_LINE_TRIGGER_SLOPE"=1250701, "ACQUISITION_SEGMENTEDMEMORY_INDEX"=1150139, "ACQUISITION_SEGMENTEDMEMORY_SEGMENT_COUNT"=1150138, "ACQUISITION_TYPE"=1250101, "CHANNEL_COUNT"=1050203, "CHANNEL_PROTECTION"=1150202, "CHANNEL_UNITS"=1150033, "DIGITALCHANNEL_COUNT"=1150038, "DIGITALCHANNEL_POSITION"=1150041, "DIGITALCHANNEL_SIZE"=1150042, "DVM_MODE"=1150443, "EXTERNAL_UNITS"=1150014, "GLITCH_CONDITION"=1250403, "GLITCH_POLARITY"=1250402, "HORZ_MIN_NUM_PTS"=1250009, "HORZ_RECORD_LENGTH"=1250008, "INTERPOLATION"=1250019, "NUM_AVERAGES"=1250104, "NUM_ENVELOPES"=1250105, "REFERENCE_SIGNAL"=1150433, "RUNT_POLARITY"=1250303, "SAMPLE_MODE"=1250106, "STATISTICS_FORMAT"=1150355, "STATUS_SERIAL_POLL"=1150019, "SYSTEM_IO_TIMEOUT"=1150607, "SYSTEM_PRECISION_RECORD_LENGTH"=1150589, "SYSTEM_TIMEOUT_MILLISECONDS"=1150023, "TIMEBASE_MODE"=1150107, "TIMEBASE_TIME_REFERENCE"=1150110, "TRIGGER_ACLINE_SLOPE"=1150556, "TRIGGER_COUPLING"=1250014, "TRIGGER_DELAY_ARMING_SLOPE"=1150263, "TRIGGER_DELAY_EDGE_COUNT"=1150267, "TRIGGER_DELAY_SLOPE"=1150266, "TRIGGER_EDGE_BURST_NTH_EDGE"=1150247, "TRIGGER_EDGE_BURST_SLOPE"=1150249, "TRIGGER_EDGE_REJECT_FILTER_TYPE"=1150135, "TRIGGER_MODIFIER"=1250102, "TRIGGER_PATTERN_CONDITION"=1150195, "TRIGGER_RUNT_CONDITION"=1150189, "TRIGGER_SETUP_AND_HOLD_SLOPE"=1150250, "TRIGGER_SLOPE"=1250018, "TRIGGER_TRANSITION_CONDITION"=1150255, "TRIGGER_TRANSITION_SLOPE"=1150256, "TRIGGER_TYPE"=1250012, "TRIGGER_TYPE_AG"=1150557, "TRIGGER_WIDTH_CONDITION"=1150197, "TRIGGER_WIDTH_POLARITY"=1150200, "VERTICAL_COUPLING"=1250003, "WAVEFORM_BYTE_ORDER"=1150085, "WAVEFORM_DATA_FORMAT"=1150086, "WAVEFORM_POINT_COUNT"=1150141, "WAVEFORM_POINT_MODE"=1150087, "WAVEFORM_SUB_SOOURCE"=1150609, "WAVEFORM_X_REFERENCE"=1150145, "WAVEFORM_Y_REFERENCE"=1150146, "WIDTH_CONDITION"=1250504, "WIDTH_POLARITY"=1250503] ("AttributeID")
  # "Turn off wavegen"
  # "waveform size maximum = 50000 -> this takes the entire waveform displayed on the oscilloscope, control is invisible on front panel"
  # "1 is edge source, would need to numbers for other source types"
  # "Enable Channels 1 & 2"
  n1 = local write "Test Type"(0) -> ()
  n2 = local write "EVENT COUNTER"(0) -> ()
  n3 = local write "SWEEP IN PROGRESS"(w28) -> ()
  n4 = local write "ACQUISITION IN PROGRESS"(w28) -> ()
  n5 = local write "PULSING IN PROGRESS"(w28) -> ()
  n6 = Concatenate Strings("File Name", ".txt") -> (w36:string)
  n7 = Build Path(base path="Save Directory", name or relative path=w36) -> (appended path=w7:path)
  "File Path" <- w7
  n8 = call <instrlib>:"Initialize.vi"("id query (Off)"=TRUE, "resource string"="Oscilloscope VISA address") -> ("error out"=w29:errorcluster, "instrument handle out"=w30:refnum<k15>)  [unwired: 8 in]
  n9 = call <instrlib>:"Reset With Defaults.vi"("error in (no error)"=w29, "instrument handle"=w30) -> ("error out"=w31:errorcluster, "instrument handle out"=w32:refnum<k15>)  [unwired: 8 in]
  n10 = call <instrlib>:"Configure Channel.vi"("channel enabled (Off)"=TRUE, "error in (no error)"=w31, "channel name"="Channel1", "instrument handle"=w32) -> ("error out"=w63:errorcluster, "instrument handle out"=w64:refnum<k15>)  [unwired: 6 in]
  n11 = call <instrlib>:"Configure Channel.vi"("channel enabled (Off)"=TRUE, "error in (no error)"=w63, "channel name"="Channel2", "instrument handle"=w64) -> ("error out"=w39:errorcluster, "instrument handle out"=w40:refnum<k15>)  [unwired: 6 in]
  n12 = call <instrlib>:"SetAttributeViReal64.vi"("AttributeValue"="Channel 1 Atten.", "error in (no error)"=w39, "AttributeID"=w69, "RepCapIdentifier"=w70, "instrument handle"=w40) -> ("error out"=w71:errorcluster, "instrument handle out"=w72:refnum<k15>)  [unwired: 5 in]
  n13 = Path To String(path=w7) -> (string=w19:string)
  n14 = call <instrlib>:"GetAttributeViReal64.vi"("error in (no error)"=w71, "AttributeID"=w69, "RepCapIdentifier"=w70, "instrument handle"=w72) -> ("error out"=w55:errorcluster, "AttributeValue"=w57:dbl, "instrument handle out"=w56:refnum<k15>)  [unwired: 5 in]
  n15 = Concatenate Strings("DalyLab_Oscilloscope_DAQ\nVersion 1.0\nJanuary 23, 2023\nN. Tulshibagwale", w22, w22, "SETUP ---------------------------------------------------------\n", "Test Operator: ", "Test Operator", w22, "VISA Address: ", "Oscilloscope VISA address", w22, "File Path: ", w19, w18, w18, "OSCILLOSCOPE CONFIGURATION  ---------------------------\n") -> (w27:string)
  n16 = Number To Fractional String(number=w57, precision (6)=i16 2) -> (F-format string=w60:string)  [unwired: 2 in]
  n17 = call <instrlib>:"SetAttributeViReal64.vi"("AttributeValue"="Channel 2 Atten.", "error in (no error)"=w55, "AttributeID"=w50, "RepCapIdentifier"=w51, "instrument handle"=w56) -> ("error out"=w53:errorcluster, "instrument handle out"=w54:refnum<k15>)  [unwired: 5 in]
  n18 = call <instrlib>:"GetAttributeViReal64.vi"("error in (no error)"=w53, "AttributeID"=w50, "RepCapIdentifier"=w51, "instrument handle"=w54) -> ("error out"=w48:errorcluster, "AttributeValue"=w42:dbl, "instrument handle out"=w49:refnum<k15>)  [unwired: 5 in]
  n19 = Concatenate Strings(w27, "Channel 1 Atten.: " ("string"), w60, "\r") -> (w43:string)
  n20 = Number To Fractional String(number=w42, precision (6)=i16 2) -> (F-format string=w46:string)  [unwired: 2 in]
  n21 = call <instrlib>:"SetAttributeViInt32.vi"("AttributeValue"=1, "error in (no error)"=w48, "AttributeID"=w188, "instrument handle"=w49) -> ("error out"=w186:errorcluster, "instrument handle out"=w185:refnum<k15>)  [unwired: 6 in]
  n22 = Concatenate Strings(w43, "Channel 2 Atten.: " ("string"), w46, "\r") -> (w21:string)
  n23 = call <instrlib>:"GetAttributeViInt32.vi"("error in (no error)"=w186, "AttributeID"=w184, "instrument handle"=w185) -> ("error out"=w177:errorcluster, "AttributeValue"=w160:i32, "instrument handle out"=w179:refnum<k15>)  [unwired: 6 in]
  n24 = property on="Trigger Edge Source" class="Ring (strict)"() -> ("RingText.Text"=w157:string)  [unwired: 2 in, 2 out]
  n25 = Number To Decimal String(number=w160) -> (decimal integer string=w169:string)  [unwired: 1 in]
  n26 = call <instrlib>:"SetAttributeViString.vi"("AttributeValue"=w157, "error in (no error)"=w177, "AttributeID"=w183, "instrument handle"=w179) -> ("error out"=w178:errorcluster, "instrument handle out"=w180:refnum<k15>)  [unwired: 6 in]
  n27 = Concatenate Strings("Trigger mode:                     " ("string"), w169, "\r") -> ()  [unwired: 1 out]
  n28 = call <instrlib>:"GetAttributeViString.vi"("AttributeValueBufferSize"=127, "error in (no error)"=w178, "AttributeID"=w182, "instrument handle"=w180) -> ("error out"=w172:errorcluster, "AttributeValue"=w159:string, "instrument handle out"=w174:refnum<k15>)  [unwired: 5 in]
  n29 = call <instrlib>:"SetAttributeViReal64.vi"("AttributeValue"="Trigger Edge Level (V)", "error in (no error)"=w172, "AttributeID"=w176, "instrument handle"=w174) -> ("error out"=w173:errorcluster, "instrument handle out"=w175:refnum<k15>)  [unwired: 6 in]
  n30 = Concatenate Strings(w21, "Trigger Edge Source: " ("AttributeValue"), w159, "\r") -> (w161:string)
  n31 = call <instrlib>:"GetAttributeViReal64.vi"("error in (no error)"=w173, "AttributeID"=w171, "instrument handle"=w175) -> ("error out"=w113:errorcluster, "AttributeValue"=w158:dbl, "instrument handle out"=w112:refnum<k15>)  [unwired: 6 in]
  n32 = Number To Fractional String(number=w158, precision (6)=i16 2) -> (F-format string=w164:string)  [unwired: 2 in]
  n33 = call <instrlib>:"SetAttributeViReal64.vi"("AttributeValue"="Channel 1 Scale (V/div)", "error in (no error)"=w113, "AttributeID"=w137, "RepCapIdentifier"=w135, "instrument handle"=w112) -> ("error out"=w133:errorcluster, "instrument handle out"=w134:refnum<k15>)  [unwired: 5 in]
  n34 = Concatenate Strings(w161, "Trigger Edge Level (V): " ("string"), w164, "\r") -> (w111:string)
  n35 = call <instrlib>:"GetAttributeViReal64.vi"("error in (no error)"=w133, "AttributeID"=w136, "RepCapIdentifier"=w135, "instrument handle"=w134) -> ("error out"=w129:errorcluster, "AttributeValue"=w110:dbl, "instrument handle out"=w128:refnum<k15>)  [unwired: 5 in]
  n36 = Number To Fractional String(number=w110, precision (6)=i16 2) -> (F-format string=w149:string)  [unwired: 2 in]
  n37 = call <instrlib>:"SetAttributeViReal64.vi"("AttributeValue"="Channel 1 Offset (V)", "error in (no error)"=w129, "AttributeID"=w132, "RepCapIdentifier"=w126, "instrument handle"=w128) -> ("error out"=w130:errorcluster, "instrument handle out"=w127:refnum<k15>)  [unwired: 5 in]
  n38 = Concatenate Strings(w111, "Channel 1 Scale (V/div): ", w149, "\r") -> (w138:string)
  n39 = call <instrlib>:"GetAttributeViReal64.vi"("error in (no error)"=w130, "AttributeID"=w131, "RepCapIdentifier"=w126, "instrument handle"=w127) -> ("error out"=w97:errorcluster, "AttributeValue"=w109:dbl, "instrument handle out"=w98:refnum<k15>)  [unwired: 5 in]
  n40 = Number To Fractional String(number=w109, precision (6)=i16 2) -> (F-format string=w150:string)  [unwired: 2 in]
  n41 = call <instrlib>:"SetAttributeViReal64.vi"("AttributeValue"="Channel 2 Scale (V/div)", "error in (no error)"=w97, "AttributeID"=w104, "RepCapIdentifier"=w102, "instrument handle"=w98) -> ("error out"=w100:errorcluster, "instrument handle out"=w101:refnum<k15>)  [unwired: 5 in]
  n42 = Concatenate Strings(w138, "Channel 1 Offset (V): ", w150, "\r") -> (w87:string)
  n43 = call <instrlib>:"GetAttributeViReal64.vi"("error in (no error)"=w100, "AttributeID"=w103, "RepCapIdentifier"=w102, "instrument handle"=w101) -> ("error out"=w79:errorcluster, "AttributeValue"=w86:dbl, "instrument handle out"=w78:refnum<k15>)  [unwired: 5 in]
  n44 = Number To Fractional String(number=w86, precision (6)=i16 2) -> (F-format string=w90:string)  [unwired: 2 in]
  n45 = call <instrlib>:"SetAttributeViReal64.vi"("AttributeValue"="Channel 2 Offset (V)", "error in (no error)"=w79, "AttributeID"=w85, "RepCapIdentifier"=w81, "instrument handle"=w78) -> ("error out"=w83:errorcluster, "instrument handle out"=w82:refnum<k15>)  [unwired: 5 in]
  n46 = Concatenate Strings(w87, "Channel 2 Scale (V/div): ", w90, "\r") -> (w88:string)
  n47 = call <instrlib>:"GetAttributeViReal64.vi"("error in (no error)"=w83, "AttributeID"=w84, "RepCapIdentifier"=w81, "instrument handle"=w82) -> ("error out"=w74:errorcluster, "AttributeValue"=w77:dbl, "instrument handle out"=w75:refnum<k15>)  [unwired: 5 in]
  n48 = Number To Fractional String(number=w77, precision (6)=i16 2) -> (F-format string=w91:string)  [unwired: 2 in]
  n49 = call <instrlib>:"SetAttributeViReal64.vi"("AttributeValue"="Horizontal Scale (s/div)", "error in (no error)"=w74, "AttributeID"=w125, "instrument handle"=w75) -> ("error out"=w124:errorcluster, "instrument handle out"=w123:refnum<k15>)  [unwired: 6 in]
  n50 = Concatenate Strings(w88, "Channel 2 Offset (V): ", w91, "\r") -> (w76:string)
  n51 = call <instrlib>:"GetAttributeViReal64.vi"("error in (no error)"=w124, "AttributeID"=w122, "instrument handle"=w123) -> ("error out"=w117:errorcluster, "AttributeValue"=w108:dbl, "instrument handle out"=w118:refnum<k15>)  [unwired: 6 in]
  n52 = Number To Fractional String(number=w108, precision (6)=i16 4) -> (F-format string=w144:string)  [unwired: 2 in]
  n53 = call <instrlib>:"SetAttributeViReal64.vi"("AttributeValue"="Acq. Start Time (s)", "error in (no error)"=w117, "AttributeID"=w121, "instrument handle"=w118) -> ("error out"=w120:errorcluster, "instrument handle out"=w73:refnum<k15>)  [unwired: 6 in]
  n54 = Concatenate Strings(w76, "Horizontal Scale (s/div): ", w144, "\r") -> (w139:string)
  n55 = call <instrlib>:"GetAttributeViReal64.vi"("error in (no error)"=w120, "AttributeID"=w119, "instrument handle"=w73) -> ("error out"=w34:errorcluster, "AttributeValue"=w107:dbl, "instrument handle out"=w35:refnum<k15>)  [unwired: 6 in]
  n56 = while {
    tunnel: w34 -> [w203]
    tunnel: w35 -> [w202]
    tunnel: [w199] -> w5
    tunnel: [w198] -> w6
    stop <- w201 stop-if-true
    # "TEST TYPE variable defined by a button push and determines the test to run, after test completion, program exits. (AE Acquisition is ended via Stop Button).\n\n1 = Pulse Generation\n2 = Acquisition\n3 = Frequency Sweep"
    # "While loop executes until user initiates a test"
    n57 = local read "Test Type"() -> (w200:i32)
    n58 = case shown="3" w200 {
      tunnel: w203 -> [w207 w222 w403 w539]
      tunnel: w202 -> [w208 w223 w402 w540]
      tunnel: [FALSE w220 w390 w533] -> w201
      tunnel: [w207 w216 w388 w529] -> w199
      tunnel: [w208 w218 w387 w530] -> w198
      frame 0, Default {
      }
      frame 1 {
        n59 = flat-sequence {
          tunnel: [w254] -> w232
          tunnel: [w255] -> w231
          tunnel: w223 -> [w250]
          tunnel: w222 -> [w249]
          tunnel: [w293] -> w230
          tunnel: [w294] -> w229
          tunnel: [w292] -> w228
          tunnel: [w291] -> w227
          tunnel: [w295] -> w226
          tunnel: w232 -> [w299]
          tunnel: w231 -> [w300]
          tunnel: w230 -> [w338]
          tunnel: w229 -> [w339]
          tunnel: w228 -> [w354]
          tunnel: [w354] -> w225
          tunnel: w227 -> [w353]
          tunnel: [w353] -> w224
          tunnel: w226 -> [w344]
          tunnel: [w339] -> w219
          tunnel: [w338] -> w217
          tunnel: w225 -> [w357]
          tunnel: w224 -> [w356]
          tunnel: [w364] -> w220
          tunnel: w219 -> [w363]
          tunnel: [w363] -> w218
          tunnel: w217 -> [w362]
          tunnel: [w362] -> w216
          frame #0 {
            w242 = u32 1150533 items=["ARBITRARY_BYTE_ORDER"=1150415, "MODULATION_FUNCTION"=1150552, "MODULATION_TYPE"=1150555, "TRACKING_PHASE"=1150659, "WAVE_GEN_ADDITIONAL_NOISE"=1150529, "WAVE_GEN_ARBITRARY_BYTE_ORDER"=1150544, "WAVE_GEN_FUNCTION"=1150533, "WAVE_GEN_OUTPUT_LOAD_IMPEDANCE"=1150538, "WAVE_GEN_OUTPUT_MODE"=1150658] ("AttributeID")
            w247 = u32 1150537 items=["ARBITRARY_INTERPOLATION"=1150411, "MODULATION_ENABLED"=1150554, "TRACKING_AMPLITUDE"=1150527, "TRACKING_ENABLED"=1150526, "TRACKING_FREQUENCY"=1150528, "WAVE_GEN_ARBITRARY_INTERPOLATION"=1150543, "WAVE_GEN_OUTPUT_ENABLED"=1150537, "WAVE_GEN_OUTPUT_INVERTED"=1150545] ("AttributeID")
            w262 = u32 1150532 items=["FM_DEVIATION"=1150548, "FM_FREQUENCY"=1150549, "FSK_FREQUENCY"=1150550, "FSK_MODULATION_RATE"=1150551, "MODULATION_RAMP_SYMMETRY"=1150553, "WAVE_GEN_AM_DEPTH"=1150546, "WAVE_GEN_AM_FREQUENCY"=1150547, "WAVE_GEN_AMPLITUDE"=1150530, "WAVE_GEN_DUTY_CYCLE"=1150531, "WAVE_GEN_FREQUENCY"=1150532, "WAVE_GEN_HIGH_VOLTAGE"=1150534, "WAVE_GEN_LOW_VOLTAGE"=1150535, "WAVE_GEN_OFFSET_VOLTAGE"=1150536, "WAVE_GEN_PERIOD"=1150539, "WAVE_GEN_PULSE_WIDTH"=1150540, "WAVE_GEN_RAMP_SYMMETRY"=1150541] ("AttributeID")
            w272 = u32 1150540 items=["FM_DEVIATION"=1150548, "FM_FREQUENCY"=1150549, "FSK_FREQUENCY"=1150550, "FSK_MODULATION_RATE"=1150551, "MODULATION_RAMP_SYMMETRY"=1150553, "WAVE_GEN_AM_DEPTH"=1150546, "WAVE_GEN_AM_FREQUENCY"=1150547, "WAVE_GEN_AMPLITUDE"=1150530, "WAVE_GEN_DUTY_CYCLE"=1150531, "WAVE_GEN_FREQUENCY"=1150532, "WAVE_GEN_HIGH_VOLTAGE"=1150534, "WAVE_GEN_LOW_VOLTAGE"=1150535, "WAVE_GEN_OFFSET_VOLTAGE"=1150536, "WAVE_GEN_PERIOD"=1150539, "WAVE_GEN_PULSE_WIDTH"=1150540, "WAVE_GEN_RAMP_SYMMETRY"=1150541] ("AttributeID")
            w259 = "\r"
            w251 = "WaveGen1" ("Measurement")
            w236 = "\r"
            w281 = u32 1150530 items=["FM_DEVIATION"=1150548, "FM_FREQUENCY"=1150549, "FSK_FREQUENCY"=1150550, "FSK_MODULATION_RATE"=1150551, "MODULATION_RAMP_SYMMETRY"=1150553, "WAVE_GEN_AM_DEPTH"=1150546, "WAVE_GEN_AM_FREQUENCY"=1150547, "WAVE_GEN_AMPLITUDE"=1150530, "WAVE_GEN_DUTY_CYCLE"=1150531, "WAVE_GEN_FREQUENCY"=1150532, "WAVE_GEN_HIGH_VOLTAGE"=1150534, "WAVE_GEN_LOW_VOLTAGE"=1150535, "WAVE_GEN_OFFSET_VOLTAGE"=1150536, "WAVE_GEN_PERIOD"=1150539, "WAVE_GEN_PULSE_WIDTH"=1150540, "WAVE_GEN_RAMP_SYMMETRY"=1150541] ("AttributeID")
            w282 = u32 1150530 items=["FM_DEVIATION"=1150548, "FM_FREQUENCY"=1150549, "FSK_FREQUENCY"=1150550, "FSK_MODULATION_RATE"=1150551, "MODULATION_RAMP_SYMMETRY"=1150553, "WAVE_GEN_AM_DEPTH"=1150546, "WAVE_GEN_AM_FREQUENCY"=1150547, "WAVE_GEN_AMPLITUDE"=1150530, "WAVE_GEN_DUTY_CYCLE"=1150531, "WAVE_GEN_FREQUENCY"=1150532, "WAVE_GEN_HIGH_VOLTAGE"=1150534, "WAVE_GEN_LOW_VOLTAGE"=1150535, "WAVE_GEN_OFFSET_VOLTAGE"=1150536, "WAVE_GEN_PERIOD"=1150539, "WAVE_GEN_PULSE_WIDTH"=1150540, "WAVE_GEN_RAMP_SYMMETRY"=1150541] ("AttributeID")
            # "3 => pulse\n\n1,2,3,4,5,6 for sine, square, etc.."
            # "Turn on wave generator and set pulse settings"
            n60 = call <instrlib>:"SetAttributeViBoolean_WAVE GEN.vi"("AttributeValue (Off)"=TRUE, "error in (no error)"=w249, "AttributeID"=w247, "instrument handle"=w250) -> ("error out"=w245:errorcluster, "instrument handle out"=w246:refnum<k15>)  [unwired: 6 in]
            n61 = call <instrlib>:"SetAttributeViInt32_WAVE GEN.vi"("AttributeValue"=3, "error in (no error)"=w245, "AttributeID"=w242, "instrument handle"=w246) -> ("error out"=w243:errorcluster, "instrument handle out"=w244:refnum<k15>)  [unwired: 6 in]
            n62 = call <instrlib>:"GetAttributeViInt32_WAVE GEN.vi"("error in (no error)"=w243, "AttributeID"=w242, "instrument handle"=w244) -> ("error out"=w240:errorcluster, "AttributeValue"=w239:i32, "instrument handle out"=w241:refnum<k15>)  [unwired: 6 in]
            n63 = call <instrlib>:"SetAttributeViReal64_WAVE GEN.vi"("AttributeValue"="Pulse Amplitude (V)", "error in (no error)"=w240, "AttributeID"=w281, "RepCapIdentifier"=w251, "instrument handle"=w241) -> ("error out"=w289:errorcluster, "instrument handle out"=w288:refnum<k15>)  [unwired: 5 in]
            n64 = call <instrlib>:"GetAttributeViReal64_WAVE GEN.vi"("error in (no error)"=w289, "AttributeID"=w282, "RepCapIdentifier"=w251, "instrument handle"=w288) -> ("error out"=w275:errorcluster, "AttributeValue"=w286:dbl, "instrument handle out"=w276:refnum<k15>)  [unwired: 5 in]
            n65 = call <instrlib>:"SetAttributeViReal64_WAVE GEN.vi"("AttributeValue"="Pulse Width (s)", "error in (no error)"=w275, "AttributeID"=w272, "RepCapIdentifier"=w251, "instrument handle"=w276) -> ("error out"=w273:errorcluster, "instrument handle out"=w274:refnum<k15>)  [unwired: 5 in]
            n66 = local read "Log"() -> (w233:string)
            n67 = Number To Decimal String(number=w239) -> (decimal integer string=w238:string)  [unwired: 1 in]
            n68 = Number To Fractional String(number=w286, precision (6)=4) -> (F-format string=w287:string)  [unwired: 2 in]
            n69 = Concatenate Strings(w233, "Waveform Type: ", w238, w236) -> ()  [unwired: 1 out]
            n70 = Concatenate Strings(w233, "Pulse Amplitude (V): ", w287, w236) -> (w280:string)
            n71 = call <instrlib>:"GetAttributeViReal64_WAVE GEN.vi"("error in (no error)"=w273, "AttributeID"=w272, "RepCapIdentifier"=w251, "instrument handle"=w274) -> ("error out"=w265:errorcluster, "AttributeValue"=w267:dbl, "instrument handle out"=w266:refnum<k15>)  [unwired: 5 in]
            n72 = Number To Decimal String(number="Number of Pulses") -> (decimal integer string=w277:string)  [unwired: 1 in]
            n73 = call <instrlib>:"SetAttributeViReal64_WAVE GEN.vi"("AttributeValue"="Rate (pulse/second)", "error in (no error)"=w265, "AttributeID"=w262, "RepCapIdentifier"=w251, "instrument handle"=w266) -> ("error out"=w263:errorcluster, "instrument handle out"=w264:refnum<k15>)  [unwired: 5 in]
            n74 = Concatenate Strings(w280, "Number of Pulses: ", w277, w259) -> (w270:string)
            n75 = call <instrlib>:"GetAttributeViReal64_WAVE GEN.vi"("error in (no error)"=w263, "AttributeID"=w262, "RepCapIdentifier"=w251, "instrument handle"=w264) -> ("error out"=w254:errorcluster, "AttributeValue"=w257:dbl, "instrument handle out"=w255:refnum<k15>)  [unwired: 5 in]
            n76 = Number To Fractional String(number=w267, precision (6)=9) -> (F-format string=w252:string)  [unwired: 2 in]
            n77 = Concatenate Strings(w270, "Pulse Width (s): ", w252, w259) -> (w261:string)
            n78 = Number To Fractional String(number=w257, precision (6)=4) -> (F-format string=w256:string)  [unwired: 2 in]
            n79 = Concatenate Strings(w261, "Rate (pulse/second): ", w256, w259) -> (w253:string)
            n80 = local write "Log"(w253) -> ()
          }
          frame #1 {
            # "When start is pressed, send pulses acquire waveform measurements for channel 1 and 2"
            # "initialize empty array for channel 1 & channel 2 waveforms"
            n81 = local read "Number of Pulses"() -> (w290:i32)
            n82 = for {
              N: w290 -> [_]
              tunnel: w300 -> [w327]
              tunnel: w299 -> [w326]
              shift-right: [w321] -> w291
              shift-left: dbl[] [] -> [w318]
              shift-right: [w320] -> w292
              shift-left: dbl[] [] -> [w319]
              tunnel: [w310] -> w294
              tunnel: [w309] -> w293
              n83 = call <instrlib>:"Initiate Acquisition.vi"("error in (no error)"=w326, "instrument handle"=w327) -> ("error out"=w316:errorcluster, "instrument handle out"=w317:refnum<k15>)  [unwired: 8 in]
              n84 = while {
                tunnel: w317 -> [w334]
                tunnel: [w333] -> w314
                tunnel: [w329] -> w315
                tunnel: w316 -> [w330]
                stop <- w328 stop-if-true
                n85 = call <instrlib>:"Acquisition Status.vi"("error in (no error)"=w330, "instrument handle"=w334) -> ("error out"=w333:errorcluster, "acquisition status"=w331:i32, "instrument handle out"=w329:refnum<k15>)  [unwired: 7 in]
                n86 = Equal?(x=w331, y=1) -> (x = y?=w328:bool)
                n87 = case shown="True" w328 {
                  frame False {
                  }
                  frame True {
                    n88 = local read "EVENT COUNTER"() -> (w335:dbl)
                    n89 = Increment(x=w335) -> (x+1=w336:dbl)
                    n90 = local write "EVENT COUNTER"(w336) -> ()
                  }
                }
              }
              n91 = local read "Waveform Size"() -> (w311:i32)
              n92 = call <instrlib>:"Measurement Fetch Waveform.vi"("error in (no error)"=w314, "WaveformSize (2048)"=w311, "Measurement"="Channel1", "instrument handle"=w315) -> ("error out"=w312:errorcluster, "WaveformArray (V)"=w322:dbl[], "instrument handle out"=w313:refnum<k15>)  [unwired: 2 in, 3 out]
              n93 = local write "Channel 1"(w322) -> ()
              n94 = Build Array (concatenate)(w318, w322) -> (w321:dbl[])
              n95 = call <instrlib>:"Measurement Fetch Waveform.vi"("error in (no error)"=w312, "WaveformSize (2048)"=w311, "Measurement"="Channel2", "instrument handle"=w313) -> ("error out"=w309:errorcluster, "WaveformArray (V)"=w323:dbl[], "instrument handle out"=w310:refnum<k15>)  [unwired: 2 in, 3 out]
              n96 = Build Array (concatenate)(w319, w323) -> (w320:dbl[])
              n97 = local write "Channel 2"(w323) -> ()
            }
            n98 = Get Date/Time String(date format (0)=2, want seconds? (F)=TRUE) -> (date string=w308:string, time string=w305:string)  [unwired: 1 in]
            n99 = call <vilib>:"Space Constant.vi"() -> ("String"=w303:string)
            n100 = local read "Log"() -> (w296:string)
            n101 = Concatenate Strings(w308, w303, w305) -> (w301:string)
            n102 = Concatenate Strings(w296, "Test Started:", w303, w301, "\r") -> (w295:string)
            n103 = local write "Log"(w295) -> ()
          }
          frame #2 {
            w340 = "\r"
            n104 = local read "EVENT COUNTER"() -> (w337:dbl)
            n105 = Get Date/Time String(date format (0)=2, want seconds? (F)=TRUE) -> (date string=w345:string, time string=w346:string)  [unwired: 1 in]
            n106 = call <vilib>:"Space Constant.vi"() -> ("String"=w342:string)
            n107 = Concatenate Strings(w345, w342, w346) -> (w341:string)
            n108 = Number To Decimal String(number=w337, width (-)=2) -> (decimal integer string=w349:string)
            n109 = Concatenate Strings(w344, "Test Ended:", w342, w341, w340, "Number of Events: ", w349, w340, w340) -> (w352:string)
            n110 = local write "Log"(w352) -> ()
          }
          frame #3 {
            w364 = TRUE
            w367 = "\r"
            # "Write header, and waveform data to file"
            n111 = local read "File Path"() -> (w359:path)
            n112 = call <vilib>:"Check if File or Folder Exists.vi"("path"=w359) -> ("file or folder exists?"=w361:bool, "dup path"=w360:path)  [unwired: 8 in, 1 out]
            n113 = case shown="True" w361 {
              tunnel: [w378 w380] -> w358
              tunnel: w360 -> [w378 w379]
              frame False {
              }
              frame True {
                n114 = Delete(path (use dialog)=w379) -> (deleted path=w380:path)  [unwired: 4 in, 2 out]
              }
            }
            n115 = Build Array(w356, w357) -> (w377:dbl[][])
            n116 = Transpose 2D Array(2D array=w377) -> (transposed array=w376:dbl[][])
            n117 = Not(x=w364) -> (.not. x?=w371:bool)
            n118 = local read "Log"() -> (w365:string)
            n119 = local write "PULSING IN PROGRESS"(w371) -> ()
            n120 = Open/Create/Replace File(file path (use dialog)=w358, operation (0:open)=T2."create", access (0:read/write)=enum16{"read/write", "read-only", "write-only"}."write-only") -> (refnum out=w373:refnum<file>)  [unwired: 3 in, 2 out]
            n121 = Concatenate Strings(w365, w367, "Ch1      Ch2 ", w367) -> (w372:string)
            n122 = Write to Text File(file (use dialog)=w373, text=w372) -> (refnum out=w370:refnum<file>)  [unwired: 2 in, 2 out]
            n123 = Close File(refnum=w370) -> (path=w369:path)  [unwired: 1 in, 1 out]
            n124 = call-poly <vilib>:"Write Delimited Spreadsheet.vi"("file path (dialog if empty)"=w369, "format (%.3f)"="%.5f", "2D data"=w376, "append to file? (new file:F)"=TRUE) -> ()  [unwired: 10 in, 2 out]
          }
        }
        n125 = local read "Log"() -> (w215:string)
        n126 = Concatenate Strings(w215, "TESTING ------------------------------------------------------\n", "Test Type: ", "Pulse Generation", "\r") -> (w210:string)
        n127 = local write "Log"(w210) -> ()
        "PULSING IN PROGRESS" <- TRUE
      }
      frame 2 {
        n128 = local read "Log"() -> (w386:string)
        n129 = Concatenate Strings(w386, "TESTING ------------------------------------------------------\n", "Test Type: ", "Acquisition", "\r") -> (w381:string)
        n130 = local write "Log"(w381) -> ()
        n131 = flat-sequence {
          tunnel: w403 -> [w422]
          tunnel: w402 -> [w421]
          tunnel: [w420] -> w401
          tunnel: [w419] -> w400
          tunnel: [w418] -> w399
          tunnel: [w415] -> w398
          tunnel: [w414] -> w397
          tunnel: [w409] -> w396
          tunnel: w401 -> [w487]
          tunnel: [w487] -> w395
          tunnel: w400 -> [w486]
          tunnel: [w486] -> w394
          tunnel: w399 -> [w485]
          tunnel: [w485] -> w393
          tunnel: w398 -> [w484]
          tunnel: [w484] -> w392
          tunnel: w397 -> [w483]
          tunnel: [w483] -> w391
          tunnel: w396 -> [w474]
          tunnel: [w508] -> w390
          tunnel: [w509] -> w387
          tunnel: [w510] -> w388
          tunnel: w395 -> [w510]
          tunnel: w394 -> [w509]
          tunnel: w393 -> [w508]
          tunnel: w392 -> [w507]
          tunnel: w391 -> [w506]
          frame #0 {
            # "When start is pressed, loop and acquire waveform measurements for channel 1 and 2 until stop button is pressed"
            # "initialize empty array"
            n132 = while {
              tunnel: w422 -> [w432]
              tunnel: w421 -> [w431]
              tunnel: [w429] -> w420
              tunnel: [w430] -> w419
              tunnel: [w424] -> w418
              shift-right: [w427] -> w415
              shift-left: dbl[] [] -> [w428]
              shift-right: [w426] -> w414
              shift-left: dbl[] [] -> [w425]
              stop <- w424 stop-if-true
              # "If stop button was not pressed, record acquired waveform"
              n133 = call <instrlib>:"Initiate Acquisition.vi"("error in (no error)"=w432, "instrument handle"=w431) -> ("error out"=w433:errorcluster, "instrument handle out"=w434:refnum<k15>)  [unwired: 8 in]
              n134 = while {
                tunnel: w433 -> [w466]
                tunnel: w434 -> [w465]
                tunnel: [w464] -> w435
                tunnel: [w463] -> w436
                tunnel: ["Stop Acquisition"] -> w424
                stop <- w460 stop-if-true
                n135 = call <instrlib>:"Acquisition Status.vi"("error in (no error)"=w466, "instrument handle"=w465) -> ("error out"=w464:errorcluster, "acquisition status"=w461:i32, "instrument handle out"=w463:refnum<k15>)  [unwired: 7 in]
                n136 = Equal?(x=w461, y=1) -> (x = y?=w459:bool)
                n137 = Or(x=w459, y="Stop Acquisition") -> (x .or. y?=w460:bool)
                n138 = Not(x="Stop Acquisition") -> (.not. x?=w457:bool)
                n139 = And(x=w457, y=w459) -> (x .and. y?=w456:bool)
                n140 = case shown="True" w456 {
                  frame False {
                  }
                  frame True {
                    n141 = local read "EVENT COUNTER"() -> (w467:dbl)
                    n142 = Increment(x=w467) -> (x+1=w468:dbl)
                    n143 = local write "EVENT COUNTER"(w468) -> ()
                  }
                }
              }
              n144 = Not(x=w424) -> (.not. x?=w423:bool)
              n145 = case shown="True" w423 {
                tunnel: w436 -> [w437 w455]
                tunnel: w435 -> [w438 w454]
                tunnel: [w437 w449] -> w430
                tunnel: [w438 w448] -> w429
                tunnel: w428 -> [w440 w447]
                tunnel: [w440 w445] -> w427
                tunnel: [w439 w443] -> w426
                tunnel: w425 -> [w439 w442]
                frame False {
                }
                frame True {
                  n146 = call <instrlib>:"Measurement Fetch Waveform.vi"("error in (no error)"=w454, "WaveformSize (2048)"="Waveform Size", "Measurement"="Channel1", "instrument handle"=w455) -> ("error out"=w450:errorcluster, "WaveformArray (V)"=w446:dbl[], "instrument handle out"=w451:refnum<k15>)  [unwired: 2 in, 3 out]
                  "Channel 1" <- w446
                  n147 = Build Array (concatenate)(w447, w446) -> (w445:dbl[])
                  n148 = call <instrlib>:"Measurement Fetch Waveform.vi"("error in (no error)"=w450, "WaveformSize (2048)"="Waveform Size", "Measurement"="Channel2", "instrument handle"=w451) -> ("error out"=w448:errorcluster, "WaveformArray (V)"=w444:dbl[], "instrument handle out"=w449:refnum<k15>)  [unwired: 2 in, 3 out]
                  "Channel 2" <- w444
                  n149 = Build Array (concatenate)(w444, w442) -> (w443:dbl[])
                }
              }
            }
            n150 = Get Date/Time String(date format (0)=2, want seconds? (F)=TRUE) -> (date string=w412:string, time string=w408:string)  [unwired: 1 in]
            n151 = call <vilib>:"Space Constant.vi"() -> ("String"=w406:string)
            n152 = Concatenate Strings(w412, w406, w408) -> (w404:string)
            n153 = local read "Log"() -> (w413:string)
            n154 = Concatenate Strings(w413, "Test Started:", w406, w404, "\r") -> (w409:string)
            n155 = local write "Log"(w409) -> ()
          }
          frame #1 {
            w470 = "\r"
            n156 = local read "EVENT COUNTER"() -> (w469:dbl)
            n157 = Get Date/Time String(date format (0)=2, want seconds? (F)=TRUE) -> (date string=w475:string, time string=w476:string)  [unwired: 1 in]
            n158 = call <vilib>:"Space Constant.vi"() -> ("String"=w472:string)
            n159 = Concatenate Strings(w475, w472, w476) -> (w471:string)
            n160 = Number To Decimal String(number=w469, width (-)=2) -> (decimal integer string=w479:string)
            n161 = Concatenate Strings(w474, "Test Ended:", w472, w471, w470, "Number of Events: ", w479, w470, w470) -> (w482:string)
            n162 = local write "Log"(w482) -> ()
          }
          frame #2 {
            w495 = "\r"
            # "Write header, and waveform data to file"
            n163 = Not(x=w508) -> (.not. x?=w499:bool)
            n164 = Build Array(w507, w506) -> (w505:dbl[][])
            n165 = local read "File Path"() -> (w490:path)
            n166 = local write "ACQUISITION IN PROGRESS"(w499) -> ()
            n167 = call <vilib>:"Check if File or Folder Exists.vi"("path"=w490) -> ("file or folder exists?"=w492:bool, "dup path"=w491:path)  [unwired: 8 in, 1 out]
            n168 = case shown="False" w492 {
              tunnel: [w511 w513] -> w489
              tunnel: w491 -> [w511 w512]
              frame False {
              }
              frame True {
                n169 = Delete(path (use dialog)=w512) -> (deleted path=w513:path)  [unwired: 4 in, 2 out]
              }
            }
            n170 = Transpose 2D Array(2D array=w505) -> (transposed array=w504:dbl[][])
            n171 = local read "Log"() -> (w493:string)
            n172 = Open/Create/Replace File(file path (use dialog)=w489, operation (0:open)=T2."create", access (0:read/write)=enum16{"read/write", "read-only", "write-only"}."write-only") -> (refnum out=w501:refnum<file>)  [unwired: 3 in, 2 out]
            n173 = Concatenate Strings(w493, w495, "Ch1      Ch2 ", w495) -> (w500:string)
            n174 = Write to Text File(file (use dialog)=w501, text=w500) -> (refnum out=w498:refnum<file>)  [unwired: 2 in, 2 out]
            n175 = Close File(refnum=w498) -> (path=w497:path)  [unwired: 1 in, 1 out]
            n176 = call-poly <vilib>:"Write Delimited Spreadsheet.vi"("file path (dialog if empty)"=w497, "format (%.3f)"="%.5f", "2D data"=w504, "append to file? (new file:F)"=TRUE) -> ()  [unwired: 10 in, 2 out]
          }
        }
        "ACQUISITION IN PROGRESS" <- TRUE
      }
      frame 3 {
        n177 = flat-sequence {
          tunnel: w540 -> [w562]
          tunnel: w539 -> [w561]
          tunnel: [w543] -> w538
          tunnel: [w542] -> w514
          tunnel: w538 -> [w588]
          tunnel: [w598] -> w536
          tunnel: [w597] -> w534
          tunnel: [w596] -> w531
          tunnel: [w595] -> w527
          tunnel: [w592] -> w519
          tunnel: [w590] -> w517
          tunnel: [w586] -> w515
          tunnel: w514 -> [w589]
          tunnel: [w701] -> w537
          tunnel: w536 -> [w701]
          tunnel: [w700] -> w535
          tunnel: w534 -> [w700]
          tunnel: [w699] -> w532
          tunnel: w531 -> [w699]
          tunnel: [w698] -> w528
          tunnel: w527 -> [w698]
          tunnel: [w695] -> w520
          tunnel: w519 -> [w695]
          tunnel: [w694] -> w518
          tunnel: w517 -> [w694]
          tunnel: [w693] -> w516
          tunnel: w515 -> [w693]
          tunnel: w537 -> [w734]
          tunnel: w535 -> [w733]
          tunnel: [w732] -> w533
          tunnel: [w731] -> w530
          tunnel: w532 -> [w731]
          tunnel: [w730] -> w529
          tunnel: w528 -> [w730]
          tunnel: w520 -> [w718]
          tunnel: w518 -> [w720]
          tunnel: w516 -> [w717]
          frame #0 {
            w546 = "\r"
            w553 = 2
            w570 = u32 1150533 items=["ARBITRARY_BYTE_ORDER"=1150415, "MODULATION_FUNCTION"=1150552, "MODULATION_TYPE"=1150555, "TRACKING_PHASE"=1150659, "WAVE_GEN_ADDITIONAL_NOISE"=1150529, "WAVE_GEN_ARBITRARY_BYTE_ORDER"=1150544, "WAVE_GEN_FUNCTION"=1150533, "WAVE_GEN_OUTPUT_LOAD_IMPEDANCE"=1150538, "WAVE_GEN_OUTPUT_MODE"=1150658] ("AttributeID")
            w575 = u32 1150537 items=["ARBITRARY_INTERPOLATION"=1150411, "MODULATION_ENABLED"=1150554, "TRACKING_AMPLITUDE"=1150527, "TRACKING_ENABLED"=1150526, "TRACKING_FREQUENCY"=1150528, "WAVE_GEN_ARBITRARY_INTERPOLATION"=1150543, "WAVE_GEN_OUTPUT_ENABLED"=1150537, "WAVE_GEN_OUTPUT_INVERTED"=1150545] ("AttributeID")
            w577 = "WaveGen1" ("Measurement")
            w564 = "\r"
            w578 = u32 1150530 items=["FM_DEVIATION"=1150548, "FM_FREQUENCY"=1150549, "FSK_FREQUENCY"=1150550, "FSK_MODULATION_RATE"=1150551, "MODULATION_RAMP_SYMMETRY"=1150553, "WAVE_GEN_AM_DEPTH"=1150546, "WAVE_GEN_AM_FREQUENCY"=1150547, "WAVE_GEN_AMPLITUDE"=1150530, "WAVE_GEN_DUTY_CYCLE"=1150531, "WAVE_GEN_FREQUENCY"=1150532, "WAVE_GEN_HIGH_VOLTAGE"=1150534, "WAVE_GEN_LOW_VOLTAGE"=1150535, "WAVE_GEN_OFFSET_VOLTAGE"=1150536, "WAVE_GEN_PERIOD"=1150539, "WAVE_GEN_PULSE_WIDTH"=1150540, "WAVE_GEN_RAMP_SYMMETRY"=1150541] ("AttributeID")
            w579 = u32 1150530 items=["FM_DEVIATION"=1150548, "FM_FREQUENCY"=1150549, "FSK_FREQUENCY"=1150550, "FSK_MODULATION_RATE"=1150551, "MODULATION_RAMP_SYMMETRY"=1150553, "WAVE_GEN_AM_DEPTH"=1150546, "WAVE_GEN_AM_FREQUENCY"=1150547, "WAVE_GEN_AMPLITUDE"=1150530, "WAVE_GEN_DUTY_CYCLE"=1150531, "WAVE_GEN_FREQUENCY"=1150532, "WAVE_GEN_HIGH_VOLTAGE"=1150534, "WAVE_GEN_LOW_VOLTAGE"=1150535, "WAVE_GEN_OFFSET_VOLTAGE"=1150536, "WAVE_GEN_PERIOD"=1150539, "WAVE_GEN_PULSE_WIDTH"=1150540, "WAVE_GEN_RAMP_SYMMETRY"=1150541] ("AttributeID")
            # "sine for type 0"
            # "Turn on wave generator and set to sine wave"
            n178 = local read "Freq. Increments (Hz)"() -> (w552:dbl)
            n179 = local read "Initial Frequency (Hz)"() -> (w558:dbl)
            n180 = local read "Stop Frequency (Hz)"() -> (w555:dbl)
            n181 = local read "Acq. per Freq."() -> (w548:i32)
            n182 = local read "Log"() -> (w544:string)
            n183 = Number To Fractional String(number=w558, precision (6)=w553) -> (F-format string=w557:string)  [unwired: 2 in]
            n184 = Number To Fractional String(number=w555, precision (6)=w553) -> (F-format string=w554:string)  [unwired: 2 in]
            n185 = Number To Fractional String(number=w552, precision (6)=w553) -> (F-format string=w551:string)  [unwired: 2 in]
            n186 = Number To Decimal String(number=w548) -> (decimal integer string=w547:string)  [unwired: 1 in]
            n187 = Concatenate Strings(w544, "Initial Frequency (Hz): ", w557, w546, "Stop Frequency (Hz): ", w554, w546, "Freq. Increments (Hz): ", w551, w546, "Acquisitions per Freq.: ", w547, w546) -> (w545:string)
            n188 = local write "Log"(w545) -> ()
            n189 = call <instrlib>:"SetAttributeViBoolean_WAVE GEN.vi"("AttributeValue (Off)"=TRUE, "error in (no error)"=w561, "AttributeID"=w575, "instrument handle"=w562) -> ("error out"=w573:errorcluster, "instrument handle out"=w574:refnum<k15>)  [unwired: 6 in]
            n190 = call <instrlib>:"SetAttributeViInt32_WAVE GEN.vi"("AttributeValue"=0, "error in (no error)"=w573, "AttributeID"=w570, "instrument handle"=w574) -> ("error out"=w571:errorcluster, "instrument handle out"=w572:refnum<k15>)  [unwired: 6 in]
            n191 = call <instrlib>:"GetAttributeViInt32_WAVE GEN.vi"("error in (no error)"=w571, "AttributeID"=w570, "instrument handle"=w572) -> ("error out"=w568:errorcluster, "AttributeValue"=w567:i32, "instrument handle out"=w569:refnum<k15>)  [unwired: 6 in]
            n192 = call <instrlib>:"SetAttributeViReal64_WAVE GEN.vi"("AttributeValue"="Amplitude (Vpp)", "error in (no error)"=w568, "AttributeID"=w578, "RepCapIdentifier"=w577, "instrument handle"=w569) -> ("error out"=w585:errorcluster, "instrument handle out"=w584:refnum<k15>)  [unwired: 5 in]
            n193 = call <instrlib>:"GetAttributeViReal64_WAVE GEN.vi"("error in (no error)"=w585, "AttributeID"=w579, "RepCapIdentifier"=w577, "instrument handle"=w584) -> ("error out"=w542:errorcluster, "AttributeValue"=w582:dbl, "instrument handle out"=w543:refnum<k15>)  [unwired: 5 in]
            n194 = Number To Decimal String(number=w567) -> (decimal integer string=w566:string)  [unwired: 1 in]
            n195 = Number To Fractional String(number=w582, precision (6)=2) -> (F-format string=w583:string)  [unwired: 2 in]
            n196 = Concatenate Strings("Waveform Type: ", w566, w564) -> ()  [unwired: 1 out]
            n197 = Concatenate Strings("Amplitude (Vpp): ", w583, w564) -> ()  [unwired: 1 out]
          }
          frame #1 {
            (unwired) dbl[] []
            # "Amplitude Ch 1"
            # "Loop through, incrementally increasing wave freq"
            # "initialize empty array"
            n198 = Get Date/Time String(date format (0)=2, want seconds? (F)=TRUE) -> (date string=w609:string, time string=w606:string)  [unwired: 1 in]
            n199 = call <vilib>:"Space Constant.vi"() -> ("String"=w604:string)
            n200 = local read "Log"() -> (w601:string)
            n201 = while {
              tunnel: [w638] -> w596
              tunnel: [w637] -> w595
              shift-right: [w639] -> w597
              shift-left: dbl[] [] -> [w641]
              shift-right: [w640] -> w598
              shift-left: dbl[] [] -> [w636]
              shift-right: [w628] -> w592
              shift-left: dbl[] [] -> [w627]
              shift-right: [w626] -> w590
              shift-left: dbl[] [] -> [w625]
              tunnel: w589 -> [w623]
              tunnel: w588 -> [w622]
              shift-right: [w611] -> w586
              shift-left: dbl[] [] -> [w610]
              i -> [w620]
              stop <- w613 stop-if-true
              # "Will the next increment be over"
              # "When start is pressed, send pulses acquire waveform measurements for channel 1 and 2"
              n202 = To Double Precision Float(number=w620) -> (double precision float=w635:dbl)
              n203 = Multiply(x="Freq. Increments (Hz)", y=w635) -> (x*y=w631:dbl)
              n204 = for {
                N: "Acq. per Freq." -> [_]
                shift-right: [w658] -> w640
                shift-left: w636 -> [w678]
                shift-right: [w680] -> w639
                shift-left: w641 -> [w679]
                tunnel: [w646] -> w638
                tunnel: [w647] -> w637
                shift-right: [w666] -> w628
                shift-left: w627 -> [w668]
                shift-right: [w664] -> w626
                shift-left: w625 -> [w663]
                tunnel: w623 -> [w662]
                tunnel: w622 -> [w661]
                shift-right: [w649] -> w611
                shift-left: w610 -> [w648]
                w644 = 50000 ("Waveform Size")
                w659 = u32 1150532 items=["FM_DEVIATION"=1150548, "FM_FREQUENCY"=1150549, "FSK_FREQUENCY"=1150550, "FSK_MODULATION_RATE"=1150551, "MODULATION_RAMP_SYMMETRY"=1150553, "WAVE_GEN_AM_DEPTH"=1150546, "WAVE_GEN_AM_FREQUENCY"=1150547, "WAVE_GEN_AMPLITUDE"=1150530, "WAVE_GEN_DUTY_CYCLE"=1150531, "WAVE_GEN_FREQUENCY"=1150532, "WAVE_GEN_HIGH_VOLTAGE"=1150534, "WAVE_GEN_LOW_VOLTAGE"=1150535, "WAVE_GEN_OFFSET_VOLTAGE"=1150536, "WAVE_GEN_PERIOD"=1150539, "WAVE_GEN_PULSE_WIDTH"=1150540, "WAVE_GEN_RAMP_SYMMETRY"=1150541] ("AttributeID")
                w651 = 15 items=["Rise Time"=0, "Fall Time"=1, "Frequency"=2, "Period"=3, "Voltage Rms"=4, "Voltage Peak To Peak"=5, "Voltage Max"=6, "Voltage Min"=7, "Voltage High"=8, "Voltage Low"=9, "Voltage Average"=10, "Width Neg"=11, "Width Pos"=12, "Duty Cycle Neg"=13, "Duty Cycle Pos"=14, "Amplitude"=15, "Voltage Cycle Rms"=16, "Voltage Cycle Average"=17, "Overshoot"=18, "Preshoot"=19, "Measurement Time At Max"=21, "Measurement Frequency Counter"=20, "Measurement Time At Min"=22, "Measurement Delay"=23, "Measurement Value At Time"=25, "Measurement Phase"=24, "Measurement Time At Value"=26, "Measurement Time Of Edge"=27, "Measurement Area"=28, "Measurement Burst Width"=29, "Measurement Falling Edge Count"=30, "Measurement Rising Edge Count"=32, "Measurement Falling Pulse Count"=31, "Measurement Rising Pulse Count"=33, "Measurement Standard Deviation"=34] ("MeasFunction (Rise Time)")
                w652 = "Channel2" ("Measurement")
                # "Delay between acquisitions, too fast and oscilloscope will crash"
                n205 = local read "Sine Freq (Hz)"() -> (w665:dbl)
                n206 = local read "Sine Freq (Hz)"() -> (w657:dbl)
                n207 = Build Array (concatenate)(w663, w665) -> (w664:dbl[])
                n208 = call <instrlib>:"SetAttributeViReal64_WAVE GEN.vi"("AttributeValue"=w657, "error in (no error)"=w662, "AttributeID"=w659, "instrument handle"=w661) -> ("error out"=w660:errorcluster, "instrument handle out"=w656:refnum<k15>)  [unwired: 6 in]
                n209 = call "Stall Data Flow.vim"("value in"=w656, "milliseconds to wait"="Delay (ms)") -> ("value out"=w655:refnum<k15>)  [unwired: 1 out]
                n210 = call <instrlib>:"Initiate Acquisition.vi"("error in (no error)"=w660, "instrument handle"=w655) -> ("error out"=w676:errorcluster, "instrument handle out"=w677:refnum<k15>)  [unwired: 8 in]
                n211 = while {
                  tunnel: w677 -> [w690]
                  tunnel: [w689] -> w674
                  tunnel: [w685] -> w675
                  tunnel: w676 -> [w686]
                  stop <- w684 stop-if-true
                  n212 = call <instrlib>:"Acquisition Status.vi"("error in (no error)"=w686, "instrument handle"=w690) -> ("error out"=w689:errorcluster, "acquisition status"=w687:i32, "instrument handle out"=w685:refnum<k15>)  [unwired: 7 in]
                  n213 = Equal?(x=w687, y=1) -> (x = y?=w684:bool)
                  n214 = case shown="True" w684 {
                    frame False {
                    }
                    frame True {
                      n215 = local read "EVENT COUNTER"() -> (w691:dbl)
                      n216 = Increment(x=w691) -> (x+1=w692:dbl)
                      n217 = local write "EVENT COUNTER"(w692) -> ()
                    }
                  }
                }
                n218 = local write "Waveform Size"(w644) -> ()
                n219 = call <instrlib>:"Measurement Fetch Waveform.vi"("error in (no error)"=w674, "WaveformSize (2048)"=w644, "Measurement"="Channel1", "instrument handle"=w675) -> ("error out"=w672:errorcluster, "WaveformArray (V)"=w681:dbl[], "instrument handle out"=w673:refnum<k15>)  [unwired: 2 in, 3 out]
                n220 = local write "Channel 1"(w681) -> ()
                n221 = Build Array (concatenate)(w678, w681) -> (w658:dbl[])
                n222 = call <instrlib>:"Measurement Fetch Waveform.vi"("error in (no error)"=w672, "WaveformSize (2048)"=w644, "Measurement"=w652, "instrument handle"=w673) -> ("error out"=w671:errorcluster, "WaveformArray (V)"=w682:dbl[], "instrument handle out"=w670:refnum<k15>)  [unwired: 2 in, 3 out]
                n223 = local write "Channel 2"(w682) -> ()
                n224 = Build Array (concatenate)(w679, w682) -> (w680:dbl[])
                n225 = call <instrlib>:"Measurement Fetch Waveform Measurement.vi"("error in (no error)"=w671, "MeasFunction (Rise Time)"=w651, "Measurement2"="Channel1" ("Measurement"), "instrument handle"=w670) -> ("error out"=w653:errorcluster, "Measurement"=w667:dbl, "instrument handle out"=w654:refnum<k15>)  [unwired: 5 in]
                n226 = Build Array (concatenate)(w668, w667) -> (w666:dbl[])
                n227 = call <instrlib>:"Measurement Fetch Waveform Measurement.vi"("error in (no error)"=w653, "MeasFunction (Rise Time)"=w651, "Measurement2"=w652, "instrument handle"=w654) -> ("error out"=w647:errorcluster, "Measurement"=w650:dbl, "instrument handle out"=w646:refnum<k15>)  [unwired: 5 in]
                n228 = Build Array (concatenate)(w648, w650) -> (w649:dbl[])
              }
              n229 = Add(x="Initial Frequency (Hz)", y=w631) -> (x+y=w624:dbl)
              n230 = Greater?(x=w624, y="Stop Frequency (Hz)") -> (0:w630:bool)
              n231 = local read "Freq. Increments (Hz)"() -> (w618:dbl)
              n232 = Not(x=w630) -> (.not. x?=w629:bool)
              n233 = Add(x=w620, y=1) -> (x+y=w619:i32)
              n234 = local read "Initial Frequency (Hz)"() -> (w616:dbl)
              n235 = case shown="True" w629 {
                tunnel: w624 -> [_ w643]
                frame False {
                }
                frame True {
                  "Sine Freq (Hz)" <- w643
                }
              }
              n236 = To Double Precision Float(number=w619) -> (double precision float=w617:dbl)
              n237 = local read "Stop Frequency (Hz)"() -> (w612:dbl)
              n238 = Multiply(x=w618, y=w617) -> (x*y=w615:dbl)
              n239 = Add(x=w616, y=w615) -> (x+y=w614:dbl)
              n240 = Greater?(x=w614, y=w612) -> (0:w613:bool)
            }
            n241 = Concatenate Strings(w609, w604, w606) -> (w602:string)
            n242 = Concatenate Strings(w601, "Test Started:", w604, w602, "\r") -> (w600:string)
            n243 = local write "Log"(w600) -> ()
          }
          frame #2 {
            w705 = "\r"
            n244 = local read "EVENT COUNTER"() -> (w696:dbl)
            n245 = Get Date/Time String(date format (0)=2, want seconds? (F)=TRUE) -> (date string=w711:string, time string=w710:string)  [unwired: 1 in]
            n246 = call <vilib>:"Space Constant.vi"() -> ("String"=w712:string)
            n247 = Concatenate Strings(w711, w712, w710) -> (w713:string)
            n248 = local read "Log"() -> (w697:string)
            n249 = Number To Decimal String(number=w696, width (-)=2) -> (decimal integer string=w709:string)
            n250 = Concatenate Strings(w697, "Test Ended:", w712, w713, w705, "Number of Events: ", w709, w705, w705) -> (w708:string)
            n251 = local write "Log"(w708) -> ()
          }
          frame #3 {
            w732 = TRUE
            (unwired) "Freq   Ch1 Amp.   Ch2 Amp."
            w729 = "\r"
            # "Entire input/output waveforms"
            # "Amplitude measurements are not written to output file, decided to output entire input/output waveforms for postprocessing instead. Left in in case, this changes due to large data amounts required by saving entire waveforms"
            # "Write header, and waveform data to file"
            n252 = Build Array(w720, w718, w717) -> (w719:dbl[][])
            n253 = Build Array(w734, w733) -> (w740:dbl[][])
            n254 = local read "File Path"() -> (w725:path)
            n255 = call <vilib>:"Check if File or Folder Exists.vi"("path"=w725) -> ("file or folder exists?"=w726:bool, "dup path"=w723:path)  [unwired: 8 in, 1 out]
            n256 = case shown="True" w726 {
              tunnel: [w741 w743] -> w724
              tunnel: w723 -> [w741 w742]
              frame False {
              }
              frame True {
                n257 = Delete(path (use dialog)=w742) -> (deleted path=w743:path)  [unwired: 4 in, 2 out]
              }
            }
            n258 = local read "Log"() -> (w735:string)
            n259 = Transpose 2D Array(2D array=w719) -> ()  [unwired: 1 out]
            n260 = Transpose 2D Array(2D array=w740) -> (transposed array=w716:dbl[][])
            n261 = Open/Create/Replace File(file path (use dialog)=w724, operation (0:open)=T2."create", access (0:read/write)=enum16{"read/write", "read-only", "write-only"}."write-only") -> (refnum out=w739:refnum<file>)  [unwired: 3 in, 2 out]
            n262 = Concatenate Strings(w735, w729, "Ch1      Ch2 ", w729) -> (w738:string)
            n263 = Not(x=w732) -> (.not. x?=w737:bool)
            n264 = local write "SWEEP IN PROGRESS"(w737) -> ()
            n265 = Write to Text File(file (use dialog)=w739, text=w738) -> (refnum out=w736:refnum<file>)  [unwired: 2 in, 2 out]
            n266 = Close File(refnum=w736) -> (path=w722:path)  [unwired: 1 in, 1 out]
            n267 = call-poly <vilib>:"Write Delimited Spreadsheet.vi"("file path (dialog if empty)"=w722, "format (%.3f)"="%.5f", "2D data"=w716, "append to file? (new file:F)"=TRUE) -> ()  [unwired: 10 in, 2 out]
          }
        }
        n268 = local read "Log"() -> (w526:string)
        n269 = Concatenate Strings(w526, "TESTING ------------------------------------------------------\n", "Test Type: ", "Frequency Sweep", "\r") -> (w522:string)
        n270 = local write "Log"(w522) -> ()
        "SWEEP IN PROGRESS" <- TRUE
      }
    }
    n271 = case shown="True" "Acquisition" {
      frame False {
      }
      frame True {
        # "Acquisition Test"
        "Test Type" <- 2
      }
    }
    n272 = case shown="True" "Pulse Generation" {
      frame False {
      }
      frame True {
        # "Pulse Generation Test"
        n273 = local write "Test Type"(1) -> ()
      }
    }
    n274 = Not(x="Acquisition") -> (.not. x?=w196:bool)
    n275 = Not(x="Pulse Generation") -> (.not. x?=w194:bool)
    n276 = And(x=w196, y=w194) -> (x .and. y?=w193:bool)
    n277 = Not(x="Frequency Sweep") -> (.not. x?=w190:bool)
    n278 = case shown="True" "Frequency Sweep" {
      frame False {
      }
      frame True {
        # "Sweep Frequencies Test"
        n279 = local write "Test Type"(3) -> ()
      }
    }
    n280 = And(x=w193, y=w190) -> (x .and. y?=w192:bool)
    n281 = case shown="True" w192 {
      frame False {
      }
      frame True {
        # "If all buttons are not pressed"
        n282 = local write "Test Type"(0) -> ()
      }
    }
  }
  n283 = Number To Fractional String(number=w107, precision (6)=i16 4) -> (F-format string=w140:string)  [unwired: 2 in]
  n284 = local read "Waveform Size"() -> (w13:i32)
  n285 = Number To Decimal String(number=w13) -> (decimal integer string=w12:string)  [unwired: 1 in]
  n286 = Concatenate Strings(w139, "Acq. Start Time (s): ", w140, "\r") -> (w11:string)
  n287 = Concatenate Strings(w11, "Waveform Size: ", w12, w9, w9) -> (→"Log":string)
  n288 = call <instrlib>:"SetAttributeViBoolean_WAVE GEN.vi"("AttributeValue (Off)"=FALSE, "error in (no error)"=w5, "AttributeID"=w2, "instrument handle"=w6) -> ("error out"=w3:errorcluster, "instrument handle out"=w4:refnum<k15>)  [unwired: 6 in]
  n289 = call <instrlib>:"Close.vi"("error in (no error)"=w3, "instrument handle"=w4) -> ()  [unwired: 9 in, 1 out]
  "EVENT COUNTER" <- 0.0
